vi "Main3.vi"() -> ()   [LabVIEW 2023]
uses:
  TEC LabVIEW Control Software v0.14/Source/LV Source/[meerstetter engineering TE Cooling]/TypeDefs/meTEC_ID 2000_Input Selection.ctl
  TEC LabVIEW Control Software v0.14/Source/LV Source/[meerstetter engineering TE Cooling]/TypeDefs/meTEC_ID 50011_Object Target Temperature Source Selection.ctl
  TEC LabVIEW Control Software v0.14/Source/LV Source/[meerstetter engineering TE Cooling]/TypeDefs/meTEC_ID 50000_Live Enable.ctl
  TEC LabVIEW Control Software v0.14/Source/LV Source/[meerstetter engineering TE Cooling]/TypeDefs/meTEC_ID 1200_Temperature is Stable.ctl
  TEC LabVIEW Control Software v0.14/Source/LV Source/[meerstetter engineering TE Cooling]/TypeDefs/meTEC_ID 104_Device Status.ctl
  Application_class/Instruments.ctl
  AD2_MSO_SDK_class/MSOConfig.ctl
  AD2_MSO_SDK_class/AD2TriggerSources.ctl
  AD2_MSO_SDK_class/MSORangeCh.ctl
  Application_class/Control 1.ctl
  Hamamatsu_class/SubRegion.ctl
  Application_class/Application.lvclass
  MTEC_Async_class/MTEC_Async.lvclass
  AD2andExtAWG_class/AD2andExtAWG.lvclass
  C:/GIT/PowerScan/InstrumentBase_class/AD2_SDK_class/InstrumentBase.lvclass
  <vilib>/Utility/error.llb/Error Cluster From Error Code.vi
  <vilib>/measure/matone.llb/Extract Single Tone Information 1 Chan.vi
  <vilib>/ErrorRing/Error Ring.xnode
  Hamamatsu_class/Hamamatsu.lvclass
  MTec_class/MTec.lvclass
  InstrumentBase_class/AD2_SDK_class/InstrumentBase.lvclass
  Experiment_class/Experiment.lvclass
  TDMSLogger_PowerScan_class/TDMSLogger_PowerScan.lvclass
  CetoniPump_class/CetoniPump.lvclass
  <vilib>/measure/NI_MAPro.lvlib
  AD2_MSO_SDK_class/AD2_MSO_SDK.lvclass
panel:
  in  "mem size":i32=100
  out "XY Graph":cluster{timestamp[], dbl[]}[](graph)=[{[timestamp(3810714974.4625654 s since 1904-01-01), timestamp(3810714974.6875706 s since 1904-01-01), timestamp(3810714974.9102407 s since 1904-01-01), timestamp(3810714975.132108 s since 1904-01-01), timestamp(3810714975.357173 s since 1904-01-01), timestamp(3810714975.581321 s since 1904-01-01), timestamp(3810714975.80342 s since 1904-01-01), timestamp(3810714976.0264726 s since 1904-01-01), timestamp(3810714976.250123 s since 1904-01-01), timestamp(3810714976.475124 s since 1904-01-01), timestamp(3810714976.6991234 s since 1904-01-01), timestamp(3810714976.9211745 s since 1904-01-01), timestamp(3810714977.1451674 s since 1904-01-01), timestamp(3810714977.368175 s since 1904-01-01), timestamp(3810714977.594176 s since 1904-01-01), timestamp(3810714977.816176 s since 1904-01-01), timestamp(3810714978.0411744 s since 1904-01-01), timestamp(3810714978.263168 s since 1904-01-01), timestamp(3810714978.488388 s since 1904-01-01), timestamp(3810714978.7113824 s since 1904-01-01), timestamp(3810714978.9333825 s since 1904-01-01), timestamp(3810714979.156552 s since 1904-01-01), timestamp(3810714979.380552 s since 1904-01-01), timestamp(3810714979.6040554 s since 1904-01-01), timestamp(3810714979.828112 s since 1904-01-01), timestamp(3810714980.051219 s since 1904-01-01), timestamp(3810714980.275273 s since 1904-01-01), timestamp(3810714980.499636 s since 1904-01-01), timestamp(3810714980.7226286 s since 1904-01-01), timestamp(3810714980.945965 s since 1904-01-01), timestamp(3810714981.170967 s since 1904-01-01), timestamp(3810714981.3933506 s since 1904-01-01), timestamp(3810714981.617357 s since 1904-01-01), timestamp(3810714981.840452 s since 1904-01-01), timestamp(3810714982.0654736 s since 1904-01-01), timestamp(3810714982.2894735 s since 1904-01-01), timestamp(3810714982.510492 s since 1904-01-01), timestamp(3810714982.734492 s since 1904-01-01), timestamp(3810714982.9584928 s since 1904-01-01), timestamp(3810714983.182848 s since 1904-01-01), timestamp(3810714983.4048495 s since 1904-01-01), timestamp(3810714983.6292033 s since 1904-01-01), timestamp(3810714983.8542337 s since 1904-01-01), timestamp(3810714984.077241 s since 1904-01-01), timestamp(3810714984.29924 s since 1904-01-01), timestamp(3810714984.52324 s since 1904-01-01), timestamp(3810714984.7462335 s since 1904-01-01), timestamp(3810714984.9702344 s since 1904-01-01), timestamp(3810714985.195372 s since 1904-01-01), timestamp(3810714985.417372 s since 1904-01-01), timestamp(3810714985.6413646 s since 1904-01-01), timestamp(3810714985.86677 s since 1904-01-01), timestamp(3810714986.0896926 s since 1904-01-01), timestamp(3810714986.311692 s since 1904-01-01), timestamp(3810714986.5356846 s since 1904-01-01), timestamp(3810714986.7598567 s since 1904-01-01), timestamp(3810714986.9828496 s since 1904-01-01), timestamp(3810714987.2071743 s since 1904-01-01), timestamp(3810714987.4291744 s since 1904-01-01), timestamp(3810714987.653329 s since 1904-01-01), timestamp(3810714987.8773217 s since 1904-01-01), timestamp(3810714988.1004457 s since 1904-01-01), timestamp(3810714988.325448 s since 1904-01-01), timestamp(3810714988.547662 s since 1904-01-01), timestamp(3810714988.7716546 s since 1904-01-01), timestamp(3810714988.994662 s since 1904-01-01), timestamp(3810714989.217661 s since 1904-01-01), timestamp(3810714989.443828 s since 1904-01-01), timestamp(3810714989.666828 s since 1904-01-01), timestamp(3810714989.890928 s since 1904-01-01), timestamp(3810714990.11292 s since 1904-01-01), timestamp(3810714990.335927 s since 1904-01-01), timestamp(3810714990.55996 s since 1904-01-01), timestamp(3810714990.7829666 s since 1904-01-01), timestamp(3810714991.006976 s since 1904-01-01), timestamp(3810714991.2310686 s since 1904-01-01), timestamp(3810714991.454176 s since 1904-01-01), timestamp(3810714991.679184 s since 1904-01-01), timestamp(3810714991.903184 s since 1904-01-01), timestamp(3810714992.125177 s since 1904-01-01), timestamp(3810714992.348177 s since 1904-01-01), timestamp(3810714992.572276 s since 1904-01-01), timestamp(3810714992.7962766 s since 1904-01-01), timestamp(3810714993.0195527 s since 1904-01-01), timestamp(3810714993.242547 s since 1904-01-01), timestamp(3810714993.4665465 s since 1904-01-01), timestamp(3810714993.6905394 s since 1904-01-01), timestamp(3810714993.913547 s since 1904-01-01), timestamp(3810714994.1385465 s since 1904-01-01), timestamp(3810714994.3625464 s since 1904-01-01), timestamp(3810714994.585547 s since 1904-01-01), timestamp(3810714994.80954 s since 1904-01-01), timestamp(3810714995.0335464 s since 1904-01-01), timestamp(3810714995.257552 s since 1904-01-01), timestamp(3810714995.4805474 s since 1904-01-01), timestamp(3810714995.7045465 s since 1904-01-01), timestamp(3810714995.925547 s since 1904-01-01), timestamp(3810714996.150547 s since 1904-01-01), timestamp(3810714996.374549 s since 1904-01-01), timestamp(3810714996.596541 s since 1904-01-01)], [22.902175903320312, 22.901992797851562, 22.903213500976562, 22.902908325195312, 22.903305053710938, 22.905197143554688, 22.906875610351562, 22.906539916992188, 22.906539916992188, 22.909378051757812, 22.910781860351562, 22.912826538085938, 22.915451049804688, 22.914047241210938, 22.917343139648438, 22.918472290039062, 22.918655395507812, 22.921981811523438, 22.920059204101562, 22.919723510742188, 22.918167114257812, 22.916549682617188, 22.915725708007812, 22.916458129882812, 22.916946411132812, 22.919662475585938, 22.916976928710938, 22.919906616210938, 22.921005249023438, 22.921249389648438, 22.922714233398438, 22.920883178710938, 22.924118041992188, 22.925735473632812, 22.928085327148438, 22.926986694335938, 22.929306030273438, 22.931716918945312, 22.930801391601562, 22.935470581054688, 22.936508178710938, 22.937179565429688, 22.939346313476562, 22.941116333007812, 22.940444946289062, 22.944534301757812, 22.943649291992188, 22.945999145507812, 22.944869995117188, 22.945846557617188, 22.945571899414062, 22.947494506835938, 22.948379516601562, 22.951004028320312, 22.948989868164062, 22.950271606445312, 22.950210571289062, 22.952072143554688, 22.951004028320312, 22.953475952148438, 22.954299926757812, 22.954116821289062, 22.953506469726562, 22.953598022460938, 22.954208374023438, 22.951828002929688, 22.953872680664062, 22.953018188476562, 22.953842163085938, 22.952865600585938, 22.955795288085938, 22.954513549804688, 22.955978393554688, 22.957351684570312, 22.954727172851562, 22.955886840820312, 22.955001831054688, 22.955825805664062, 22.954360961914062, 22.955032348632812, 22.957229614257812, 22.955490112304688, 22.958755493164062, 22.959518432617188, 22.959548950195312, 22.956710815429688, 22.959915161132812, 22.959487915039062, 22.959426879882812, 22.960617065429688, 22.960525512695312, 22.959243774414062, 22.960983276367188, 22.960647583007812, 22.962112426757812, 22.964004516601562, 22.964279174804688, 22.965377807617188, 22.964614868164062, 22.965621948242188]}, {[timestamp(3810714974.4625654 s since 1904-01-01), timestamp(3810714974.6875706 s since 1904-01-01), timestamp(3810714974.9102407 s since 1904-01-01), timestamp(3810714975.132108 s since 1904-01-01), timestamp(3810714975.357173 s since 1904-01-01), timestamp(3810714975.581321 s since 1904-01-01), timestamp(3810714975.80342 s since 1904-01-01), timestamp(3810714976.0264726 s since 1904-01-01), timestamp(3810714976.250123 s since 1904-01-01), timestamp(3810714976.475124 s since 1904-01-01), timestamp(3810714976.6991234 s since 1904-01-01), timestamp(3810714976.9211745 s since 1904-01-01), timestamp(3810714977.1451674 s since 1904-01-01), timestamp(3810714977.368175 s since 1904-01-01), timestamp(3810714977.594176 s since 1904-01-01), timestamp(3810714977.816176 s since 1904-01-01), timestamp(3810714978.0411744 s since 1904-01-01), timestamp(3810714978.263168 s since 1904-01-01), timestamp(3810714978.488388 s since 1904-01-01), timestamp(3810714978.7113824 s since 1904-01-01), timestamp(3810714978.9333825 s since 1904-01-01), timestamp(3810714979.156552 s since 1904-01-01), timestamp(3810714979.380552 s since 1904-01-01), timestamp(3810714979.6040554 s since 1904-01-01), timestamp(3810714979.828112 s since 1904-01-01), timestamp(3810714980.051219 s since 1904-01-01), timestamp(3810714980.275273 s since 1904-01-01), timestamp(3810714980.499636 s since 1904-01-01), timestamp(3810714980.7226286 s since 1904-01-01), timestamp(3810714980.945965 s since 1904-01-01), timestamp(3810714981.170967 s since 1904-01-01), timestamp(3810714981.3933506 s since 1904-01-01), timestamp(3810714981.617357 s since 1904-01-01), timestamp(3810714981.840452 s since 1904-01-01), timestamp(3810714982.0654736 s since 1904-01-01), timestamp(3810714982.2894735 s since 1904-01-01), timestamp(3810714982.510492 s since 1904-01-01), timestamp(3810714982.734492 s since 1904-01-01), timestamp(3810714982.9584928 s since 1904-01-01), timestamp(3810714983.182848 s since 1904-01-01), timestamp(3810714983.4048495 s since 1904-01-01), timestamp(3810714983.6292033 s since 1904-01-01), timestamp(3810714983.8542337 s since 1904-01-01), timestamp(3810714984.077241 s since 1904-01-01), timestamp(3810714984.29924 s since 1904-01-01), timestamp(3810714984.52324 s since 1904-01-01), timestamp(3810714984.7462335 s since 1904-01-01), timestamp(3810714984.9702344 s since 1904-01-01), timestamp(3810714985.195372 s since 1904-01-01), timestamp(3810714985.417372 s since 1904-01-01), timestamp(3810714985.6413646 s since 1904-01-01), timestamp(3810714985.86677 s since 1904-01-01), timestamp(3810714986.0896926 s since 1904-01-01), timestamp(3810714986.311692 s since 1904-01-01), timestamp(3810714986.5356846 s since 1904-01-01), timestamp(3810714986.7598567 s since 1904-01-01), timestamp(3810714986.9828496 s since 1904-01-01), timestamp(3810714987.2071743 s since 1904-01-01), timestamp(3810714987.4291744 s since 1904-01-01), timestamp(3810714987.653329 s since 1904-01-01), timestamp(3810714987.8773217 s since 1904-01-01), timestamp(3810714988.1004457 s since 1904-01-01), timestamp(3810714988.325448 s since 1904-01-01), timestamp(3810714988.547662 s since 1904-01-01), timestamp(3810714988.7716546 s since 1904-01-01), timestamp(3810714988.994662 s since 1904-01-01), timestamp(3810714989.217661 s since 1904-01-01), timestamp(3810714989.443828 s since 1904-01-01), timestamp(3810714989.666828 s since 1904-01-01), timestamp(3810714989.890928 s since 1904-01-01), timestamp(3810714990.11292 s since 1904-01-01), timestamp(3810714990.335927 s since 1904-01-01), timestamp(3810714990.55996 s since 1904-01-01), timestamp(3810714990.7829666 s since 1904-01-01), timestamp(3810714991.006976 s since 1904-01-01), timestamp(3810714991.2310686 s since 1904-01-01), timestamp(3810714991.454176 s since 1904-01-01), timestamp(3810714991.679184 s since 1904-01-01), timestamp(3810714991.903184 s since 1904-01-01), timestamp(3810714992.125177 s since 1904-01-01), timestamp(3810714992.348177 s since 1904-01-01), timestamp(3810714992.572276 s since 1904-01-01), timestamp(3810714992.7962766 s since 1904-01-01), timestamp(3810714993.0195527 s since 1904-01-01), timestamp(3810714993.242547 s since 1904-01-01), timestamp(3810714993.4665465 s since 1904-01-01), timestamp(3810714993.6905394 s since 1904-01-01), timestamp(3810714993.913547 s since 1904-01-01), timestamp(3810714994.1385465 s since 1904-01-01), timestamp(3810714994.3625464 s since 1904-01-01), timestamp(3810714994.585547 s since 1904-01-01), timestamp(3810714994.80954 s since 1904-01-01), timestamp(3810714995.0335464 s since 1904-01-01), timestamp(3810714995.257552 s since 1904-01-01), timestamp(3810714995.4805474 s since 1904-01-01), timestamp(3810714995.7045465 s since 1904-01-01), timestamp(3810714995.925547 s since 1904-01-01), timestamp(3810714996.150547 s since 1904-01-01), timestamp(3810714996.374549 s since 1904-01-01), timestamp(3810714996.596541 s since 1904-01-01)], [23.093063354492188, 23.094924926757812, 23.094497680664062, 23.097518920898438, 23.095504760742188, 23.094528198242188, 23.098098754882812, 23.099533081054688, 23.102035522460938, 23.100082397460938, 23.105026245117188, 23.107894897460938, 23.107254028320312, 23.108169555664062, 23.112472534179688, 23.110580444335938, 23.116165161132812, 23.113418579101562, 23.113418579101562, 23.112075805664062, 23.110916137695312, 23.108871459960938, 23.107559204101562, 23.110641479492188, 23.111648559570312, 23.111618041992188, 23.113174438476562, 23.115737915039062, 23.115188598632812, 23.116897583007812, 23.113906860351562, 23.116683959960938, 23.119857788085938, 23.119705200195312, 23.120559692382812, 23.123886108398438, 23.123031616210938, 23.122512817382812, 23.124221801757812, 23.128158569335938, 23.127243041992188, 23.129959106445312, 23.131637573242188, 23.131820678710938, 23.133285522460938, 23.136337280273438, 23.136276245117188, 23.136917114257812, 23.138320922851562, 23.137313842773438, 23.141921997070312, 23.142196655273438, 23.142440795898438, 23.143112182617188, 23.145858764648438, 23.144485473632812, 23.147598266601562, 23.147171020507812, 23.149276733398438, 23.149337768554688, 23.149276733398438, 23.152023315429688, 23.155258178710938, 23.155410766601562, 23.153366088867188, 23.155471801757812, 23.154800415039062, 23.155899047851562, 23.157669067382812, 23.159255981445312, 23.157211303710938, 23.157821655273438, 23.160781860351562, 23.162673950195312, 23.161300659179688, 23.164657592773438, 23.164108276367188, 23.163711547851562, 23.162490844726562, 23.165390014648438, 23.165481567382812, 23.165939331054688, 23.165573120117188, 23.169692993164062, 23.168869018554688, 23.167984008789062, 23.168258666992188, 23.168411254882812, 23.168258666992188, 23.168899536132812, 23.170425415039062, 23.170089721679688, 23.171829223632812, 23.173904418945312, 23.172744750976562, 23.175460815429688, 23.173141479492188, 23.174606323242188, 23.174728393554688, 23.175674438476562]}, {[timestamp(3810714974.4625654 s since 1904-01-01), timestamp(3810714974.6875706 s since 1904-01-01), timestamp(3810714974.9102407 s since 1904-01-01), timestamp(3810714975.132108 s since 1904-01-01), timestamp(3810714975.357173 s since 1904-01-01), timestamp(3810714975.581321 s since 1904-01-01), timestamp(3810714975.80342 s since 1904-01-01), timestamp(3810714976.0264726 s since 1904-01-01), timestamp(3810714976.250123 s since 1904-01-01), timestamp(3810714976.475124 s since 1904-01-01), timestamp(3810714976.6991234 s since 1904-01-01), timestamp(3810714976.9211745 s since 1904-01-01), timestamp(3810714977.1451674 s since 1904-01-01), timestamp(3810714977.368175 s since 1904-01-01), timestamp(3810714977.594176 s since 1904-01-01), timestamp(3810714977.816176 s since 1904-01-01), timestamp(3810714978.0411744 s since 1904-01-01), timestamp(3810714978.263168 s since 1904-01-01), timestamp(3810714978.488388 s since 1904-01-01), timestamp(3810714978.7113824 s since 1904-01-01), timestamp(3810714978.9333825 s since 1904-01-01), timestamp(3810714979.156552 s since 1904-01-01), timestamp(3810714979.380552 s since 1904-01-01), timestamp(3810714979.6040554 s since 1904-01-01), timestamp(3810714979.828112 s since 1904-01-01), timestamp(3810714980.051219 s since 1904-01-01), timestamp(3810714980.275273 s since 1904-01-01), timestamp(3810714980.499636 s since 1904-01-01), timestamp(3810714980.7226286 s since 1904-01-01), timestamp(3810714980.945965 s since 1904-01-01), timestamp(3810714981.170967 s since 1904-01-01), timestamp(3810714981.3933506 s since 1904-01-01), timestamp(3810714981.617357 s since 1904-01-01), timestamp(3810714981.840452 s since 1904-01-01), timestamp(3810714982.0654736 s since 1904-01-01), timestamp(3810714982.2894735 s since 1904-01-01), timestamp(3810714982.510492 s since 1904-01-01), timestamp(3810714982.734492 s since 1904-01-01), timestamp(3810714982.9584928 s since 1904-01-01), timestamp(3810714983.182848 s since 1904-01-01), timestamp(3810714983.4048495 s since 1904-01-01), timestamp(3810714983.6292033 s since 1904-01-01), timestamp(3810714983.8542337 s since 1904-01-01), timestamp(3810714984.077241 s since 1904-01-01), timestamp(3810714984.29924 s since 1904-01-01), timestamp(3810714984.52324 s since 1904-01-01), timestamp(3810714984.7462335 s since 1904-01-01), timestamp(3810714984.9702344 s since 1904-01-01), timestamp(3810714985.195372 s since 1904-01-01), timestamp(3810714985.417372 s since 1904-01-01), timestamp(3810714985.6413646 s since 1904-01-01), timestamp(3810714985.86677 s since 1904-01-01), timestamp(3810714986.0896926 s since 1904-01-01), timestamp(3810714986.311692 s since 1904-01-01), timestamp(3810714986.5356846 s since 1904-01-01), timestamp(3810714986.7598567 s since 1904-01-01), timestamp(3810714986.9828496 s since 1904-01-01), timestamp(3810714987.2071743 s since 1904-01-01), timestamp(3810714987.4291744 s since 1904-01-01), timestamp(3810714987.653329 s since 1904-01-01), timestamp(3810714987.8773217 s since 1904-01-01), timestamp(3810714988.1004457 s since 1904-01-01), timestamp(3810714988.325448 s since 1904-01-01), timestamp(3810714988.547662 s since 1904-01-01), timestamp(3810714988.7716546 s since 1904-01-01), timestamp(3810714988.994662 s since 1904-01-01), timestamp(3810714989.217661 s since 1904-01-01), timestamp(3810714989.443828 s since 1904-01-01), timestamp(3810714989.666828 s since 1904-01-01), timestamp(3810714989.890928 s since 1904-01-01), timestamp(3810714990.11292 s since 1904-01-01), timestamp(3810714990.335927 s since 1904-01-01), timestamp(3810714990.55996 s since 1904-01-01), timestamp(3810714990.7829666 s since 1904-01-01), timestamp(3810714991.006976 s since 1904-01-01), timestamp(3810714991.2310686 s since 1904-01-01), timestamp(3810714991.454176 s since 1904-01-01), timestamp(3810714991.679184 s since 1904-01-01), timestamp(3810714991.903184 s since 1904-01-01), timestamp(3810714992.125177 s since 1904-01-01), timestamp(3810714992.348177 s since 1904-01-01), timestamp(3810714992.572276 s since 1904-01-01), timestamp(3810714992.7962766 s since 1904-01-01), timestamp(3810714993.0195527 s since 1904-01-01), timestamp(3810714993.242547 s since 1904-01-01), timestamp(3810714993.4665465 s since 1904-01-01), timestamp(3810714993.6905394 s since 1904-01-01), timestamp(3810714993.913547 s since 1904-01-01), timestamp(3810714994.1385465 s since 1904-01-01), timestamp(3810714994.3625464 s since 1904-01-01), timestamp(3810714994.585547 s since 1904-01-01), timestamp(3810714994.80954 s since 1904-01-01), timestamp(3810714995.0335464 s since 1904-01-01), timestamp(3810714995.257552 s since 1904-01-01), timestamp(3810714995.4805474 s since 1904-01-01), timestamp(3810714995.7045465 s since 1904-01-01), timestamp(3810714995.925547 s since 1904-01-01), timestamp(3810714996.150547 s since 1904-01-01), timestamp(3810714996.374549 s since 1904-01-01), timestamp(3810714996.596541 s since 1904-01-01)], [0.0, 0.0, 0.0, 0.0, 0.0, 0.0, 0.0, 0.0, 0.0, 0.0, 0.0, 0.0, 0.0, 0.0, 0.0, 0.0, 0.0, 0.0, 0.0, 0.0, 0.0, 0.0, 0.0, 0.0, 0.0, 0.0, 0.0, 0.0, 0.0, 0.0, 0.0, 0.0, 0.0, 0.0, 0.0, 0.0, 0.0, 0.0, 0.0, 0.0, 0.0, 0.0, 0.0, 0.0, 0.0, 0.0, 0.0, 0.0, 0.0, 0.0, 0.0, 0.0, 0.0, 0.0, 0.0, 0.0, 0.0, 0.0, 0.0, 0.0, 0.0, 0.0, 0.0, 0.0, 0.0, 0.0, 0.0, 0.0, 0.0, 0.0, 0.0, 0.0, 0.0, 0.0, 0.0, 0.0, 0.0, 0.0, 0.0, 0.0, 0.0, 0.0, 0.0, 0.0, 0.0, 0.0, 0.0, 0.0, 0.0, 0.0, 0.0, 0.0, 0.0, 0.0, 0.0, 0.0, 0.0, 0.0, 0.0, 0.0]}]
  in  "Chart Length":enum16{"60 s", "10 minutes", "1 h"}(ring)=enum."10 minutes"
  out "Waveform Chart":waveform(dbl)[](graph)=[{"t0"=timestamp(3810714996.596541 s since 1904-01-01), "dt"=1.0, "Y"=[22.965621948242188]}, {"t0"=timestamp(3810714996.596541 s since 1904-01-01), "dt"=1.0, "Y"=[23.175674438476562]}]
  in  "Read MSO":bool
  out "error out":errorcluster
  out "Status":string="Exiting.."
  in  "AutoScaleCh1":bool=TRUE caption="AutoScale timebase to ChA"
  out "V/Hz/Deg":dbl[](array[numeric])=[256495.2123849432, 0.012104949851784449, 127.31074154871095, 4268838.632377055, 0.0003381910830981614, 134.9693104826537]
  out "Data":string[](array[string])=["Ch1Freq", "Ch1Amp", "Ch1Phase", "Ch2Freq", "Ch2Amp", "Ch2Phase"]
  out "MSO Data WaveForms 2":waveform(dbl)[](graph)=[{"t0"=timestamp(0 s since 1904-01-01), "dt"=1e-08, "Y"=array[8192 elements]}, {"t0"=timestamp(0 s since 1904-01-01), "dt"=1e-08, "Y"=array[8192 elements]}]
  in  "ABORT":bool
  in  "Tab Control":T1(tab)=enum."Cetoni"
  in  "Use Cetoni?":bool=TRUE
  in  "Use Hamamatsu":bool=TRUE
  in  "Use MeTEC?":bool=TRUE
  in  "AWG VISA resource name":refnum<visa-resource-name>="USB0::0x0699::0x0347::C037907::INSTR"
  in  "System Configuration":T2
  in  "Initialize System":bool
  in  "Use Instruments?":bool=TRUE
  in  "Device Configuration Path":string="C:\\Users\\Public\\Documents\\QmixElements\\Projects\\default_project\\Configurations\\double"
  in  "Turn Off WFG During Refill":bool
  in  "index":i32
  in  "refill below level(uL)":dbl=1000.0
  in  "Refill":bool
  in  "Conditional Refill":bool
  in  "Empty":bool
  in  "Stop pumps":bool
  in  "SyringeSettings":T3={"Maximum Piston Stroke (mm)"=66.0, "Inner Diameter (mm)"=14.5}
  in  "Configure Syringe":bool
  in  "ValveControl":cluster{"index":i32, "Valve Position":bool}
  in  "Go to Level":bool
  in  "GoToLevelSettings":T4={"index"=0, "Level(uL)"=0.0, "Flow"=250.0}
  in  "Monitor Pump":bool
  out "Array":T5(array[cluster])=[{"Pump Name"="neMESYS_Low_Pressure_1_Pump", "Actual Flow Rate"=249.9994261659258, "Fill Level"=9609.141943854513, "Is pumping"=TRUE}, {"Pump Name"="neMESYS_Low_Pressure_2_Pump", "Actual Flow Rate"=0.0, "Fill Level"=0.0, "Is pumping"=FALSE}]
  in  "ReferenceMove":bool
  in  "refill and \nempty rate(uL/min)":dbl=12000.0
  out "Cluster":T8={"meTEC_CH2_Temperature Stability"=0, "meTEC_CH2_Act. Output Current [A]"=0.009997940622270107, "meTEC_CH2_Act. Output Voltage [V]"=0.004072710871696472, "meTEC_CH2_Object Temperature [°C]"=23.175674438476562, "meTEC_CH2_Sink Temperature [°C]"=25.0, "meTEC_CH1_Error Parameter"=0, "meTEC_CH1_Error Instance"=0, "meTEC_CH1_Error No."=0, "meTEC_CH1_Device Status"=1, "meTEC_CH1_Temperature Stability"=0, "meTEC_CH1_Act. Output Current [A]"=0.010120010934770107, "meTEC_CH1_Act. Output Voltage [V]"=0.009891997091472149, "meTEC_CH1_Object Temperature [°C]"=22.965621948242188, "meTEC_CH1_Sink Temperature [°C]"=25.0} {"meTEC_CH1_Sink Temperature [°C]" format="%.3f"; "meTEC_CH1_Object Temperature [°C]" format="%.3f"; "meTEC_CH1_Act. Output Voltage [V]" format="%.3f"; "meTEC_CH1_Act. Output Current [A]" format="%.3f"; "meTEC_CH1_Temperature Stability" items=["Temperature regulation is not active", "Is not stable", "Is stable"]; "meTEC_CH1_Device Status" items=["Initializing", "Ready", "Run", "Error", "Bootloader", "Reset in Progress"]; "meTEC_CH2_Sink Temperature [°C]" format="%.3f"; "meTEC_CH2_Object Temperature [°C]" format="%.3f"; "meTEC_CH2_Act. Output Voltage [V]" format="%.3f"; "meTEC_CH2_Act. Output Current [A]" format="%.3f"; "meTEC_CH2_Temperature Stability" items=["Temperature regulation is not active", "Is not stable", "Is stable"]}
  in  "Config Data":T12={"meTEC_CH1_Input Selection (ID 2000)"=2, "meTEC_CH2_Input Selection (ID 2000)"=2, "meTEC_CH1_Object Target Temp. Source Selection (ID 50011)"=0, "meTEC_CH2_Object Target Temp. Source Selection (ID 50011)"=0, "meTEC_CH1_Live Enable (ID 50000)"=0, "meTEC_CH2_Live Enable (ID 50000)"=0, "meTEC_CH1_Object Target Temperature (ID 3000 / 50012) [°C]"=23.0, "meTEC_CH2_Object Target Temperature (ID 3000 / 50012) [°C]"=23.0, "meTEC_CH1_Live Set Current (ID 50001) [A]"=0.0, "meTEC_CH2_Live Set Current (ID 50001) [A]"=0.0, "meTEC_CH1_Live Set Voltage (ID 50002) [V]"=0.0, "meTEC_CH2_Live Set Voltage (ID 50002) [V]"=0.0} {"meTEC_CH2_Live Set Voltage (ID 50002) [V]" format="%#.3f"; "meTEC_CH1_Live Set Voltage (ID 50002) [V]" format="%#.3f"; "meTEC_CH2_Live Set Current (ID 50001) [A]" format="%#.3f"; "meTEC_CH1_Live Set Current (ID 50001) [A]" format="%#.3f"; "meTEC_CH2_Object Target Temperature (ID 3000 / 50012) [°C]" format="%#.3f"; "meTEC_CH1_Object Target Temperature (ID 3000 / 50012) [°C]" format="%#.3f"; "meTEC_CH2_Live Enable (ID 50000)" items=["Disabled (Reset State)", "Enabled"]; "meTEC_CH1_Live Enable (ID 50000)" items=["Disabled (Reset State)", "Enabled"]; "meTEC_CH2_Object Target Temp. Source Selection (ID 50011)" items=["Parameter ID 3000 (Reset State)", "Parameter ID 50012"]; "meTEC_CH1_Object Target Temp. Source Selection (ID 50011)" items=["Parameter ID 3000 (Reset State)", "Parameter ID 50012"]; "meTEC_CH2_Input Selection (ID 2000)" items=["Static Current / Voltage", "Live Current / Voltage", "Temperature Controller"]; "meTEC_CH1_Input Selection (ID 2000)" items=["Static Current / Voltage", "Live Current / Voltage", "Temperature Controller"]}
  in  "Configure TEC":bool
  in  "Monitor":bool=TRUE
  in  "ResetMtec":bool
  in  "Metec Flush Memory":bool
  in  "OutputEnable":T13
  in  "Config WFG":bool
  in  "Freq Ch1&2":T14
  in  "Configdatastd":T15={"ConfigDataCh1"={"Frequency Hz (1000 Hz)"=1000.0, "Waveform Function (0: Sine)"=0, "Amplitude (1 Vpp)"=1.0, "DC Offset (0.00 V)"=0.0, "Phase Level (-1)"=0.0, "Phase Unit (0: Radian)"=0}, "ConfigDataCh2"={"Frequency Hz (1000 Hz)"=1000.0, "Waveform Function (0: Sine)"=0, "Amplitude (1 Vpp)"=1.0, "DC Offset (0.00 V)"=0.0, "Phase Level (-1)"=0.0, "Phase Unit (0: Radian)"=0}} {"ConfigDataCh1"."Frequency Hz (1000 Hz)" min=0.0 max=100000000.0}
  in  "CurrentProbeScaling(V/A)":dbl=5.0
  in  "PwrScanSettings":T16={"FreqStart(Hz)"=1800000.0, "Increment(Hz)"=1000.0, "Steps"=100}
  out "Power Graph":T17=[{"PwrFreq"=[1800000.0, 1801000.0, 1802000.0, 1803000.0, 1804000.0, 1805000.0, 1806000.0, 1807000.0, 1808000.0, 1809000.0, 1810000.0, 1811000.0, 1812000.0, 1813000.0, 1814000.0, 1815000.0, 1816000.0, 1817000.0, 1818000.0, 1819000.0, 1820000.0, 1821000.0, 1822000.0, 1823000.0, 1824000.0, 1825000.0, 1826000.0, 1827000.0, 1828000.0, 1829000.0, 1830000.0, 1831000.0, 1832000.0, 1833000.0, 1834000.0, 1835000.0, 1836000.0, 1837000.0, 1838000.0, 1839000.0, 1840000.0, 1841000.0, 1842000.0, 1843000.0, 1844000.0, 1845000.0, 1846000.0, 1847000.0, 1848000.0, 1849000.0, 1850000.0, 1851000.0, 1852000.0, 1853000.0, 1854000.0, 1855000.0, 1856000.0, 1857000.0, 1858000.0, 1859000.0, 1860000.0, 1861000.0, 1862000.0, 1863000.0, 1864000.0, 1865000.0, 1866000.0, 1867000.0, 1868000.0, 1869000.0, 1870000.0, 1871000.0, 1872000.0, 1873000.0, 1874000.0, 1875000.0, 1876000.0, 1877000.0, 1878000.0, 1879000.0, 1880000.0, 1881000.0, 1882000.0, 1883000.0, 1884000.0, 1885000.0, 1886000.0, 1887000.0, 1888000.0, 1889000.0, 1890000.0, 1891000.0, 1892000.0, 1893000.0, 1894000.0, 1895000.0, 1896000.0, 1897000.0, 1898000.0, 1899000.0], "PwrMeasured"=[0.03743018699905172, 0.03868842711054406, 0.039939450983681936, 0.041186940846945984, 0.042492363236693975, 0.04404846555067622, 0.04602835102242353, 0.04843888820937301, 0.05119026075250401, 0.054137745072059686, 0.05681989848669318, 0.05866977349663312, 0.05974650294953525, 0.06005376515825572, 0.05994285605916934, 0.05965859181003201, 0.05940789816848652, 0.05911436810870655, 0.05887115083576992, 0.058285278937152116, 0.05733209401753114, 0.05612065814579392, 0.05491201122450486, 0.054246204884069796, 0.05413387963390649, 0.0544784492868222, 0.055223443274043806, 0.05584761484864832, 0.05593777472478643, 0.055604310692913786, 0.05518644597062401, 0.054618464862787694, 0.054214223715299915, 0.05394256784700533, 0.0538322569007853, 0.05378224385812821, 0.053684397213232725, 0.053570515853526054, 0.05367988225271155, 0.05367731285637497, 0.05328103475935342, 0.05261733484260826, 0.05172095371283941, 0.050922021343682664, 0.05021598202266246, 0.049693559571941236, 0.04964157824916153, 0.049770317527984026, 0.04982229343352004, 0.0491940448801376, 0.048088239496034246, 0.0465169483544214, 0.0449815088404273, 0.04339710247015175, 0.04200318845517933, 0.04079371088999795, 0.03986802195324547, 0.038792483453571246, 0.03777766173772913, 0.03677527534117768, 0.0359760414327305, 0.03518671210489007, 0.03475002270949958, 0.03471532342952112, 0.03517735874853088, 0.03613562839997322, 0.0377065106935801, 0.0398207089338458, 0.04192610453201364, 0.04433368155489899, 0.04724045693183674, 0.05041187326865423, 0.05357414254285915, 0.056935687754456586, 0.06034831631771629, 0.06370638524387114, 0.06689701401467622, 0.06907501466358135, 0.07011171729016413, 0.06928919978057443, 0.06697831206028507, 0.06356111518422408, 0.059707919276213384, 0.055820271940164715, 0.05201579594450088, 0.048220123240964884, 0.044549547433591366, 0.04117661978432694, 0.038128405762736364, 0.03561051707739825, 0.03331342696116638, 0.03141526136270806, 0.029497507637866037, 0.02786984120696333, 0.0266553633197663, 0.025619681037449903, 0.024768741920820493, 0.024028995090048973, 0.023324807778494015, 0.022671870223729386]}, {"PwrFreq"=[], "PwrMeasured"=[]}, {"PwrFreq"=[], "PwrMeasured"=[]}]
  in  "AdjustPower":bool
  in  "DesiredPower(W)":dbl=0.001 min=0.001
  out "min Power":dbl=0.022671870223729386
  out "max Power":dbl=0.07011171729016413
  out "Measured Power":dbl=0.014358194668451557
  in  "MeasurePower":bool
  out "AmplitudeOk":bool=TRUE
  in  "Run Power Scan":bool
  out "phase (deg)":dbl=82.9743375382008
  out "impedance (ohm)":dbl=0.07240014859741192
  in  "Config":T18={"Timing"={"Enable"=TRUE, "Samples In"=8000.0, "Sample Rate"=100000000.0, "Mode"=enum."Single Sample"}, "Trigger"={"Hysteresis"=0.0, "Trigger Level"=0.0, "Trigger Condition"=0, "Trigger Type"=0, "Trigger Channel"=0, "secTimeout"=0.5, "TrigrSrc"=enum."trigsrcDetectorAnalogIn"}, "Range Ch1"={"idxChannel"=0, "voltOffset"=0.0, "VoltsRange"=50}, "Range Ch 2"={"idxChannel"=1, "voltOffset"=0.0, "VoltsRange"=5}} {"Range Ch 2"."VoltsRange" items=["High 50V"=50, "Low5V"=5]; "Range Ch1"."VoltsRange" items=["High 50V"=50, "Low5V"=5]; "Trigger"."Trigger Channel" items=["Channel 1"=0, "Channel 2"=1, "Both"=-1]; "Trigger"."Trigger Type" items=["Edge", "Pulse", "Transition"]; "Trigger"."Trigger Condition" items=["Rising", "Falling"]}
  in  "Configure MSO":bool
  in  "AutoRange MSO (Volt)":bool
  in  "Center ROI":bool=TRUE
  in  "Image":bool
  in  "Image Continous":bool
  in  "ExposureTime(ms)":dbl=5.0
  in  "ROI":T21={"Horizontal Offset"=0, "Vertical Offset"=652, "Horizontal Size"=2304, "Vertical Size"=1000} {"Vertical Size" min=4 max=1652 step=4; "Horizontal Size" min=4 max=2304 step=4; "Vertical Offset" min=0 max=1304 step=4; "Horizontal Offset" min=0 max=0 step=4}
  in  "Configure":bool
  in  "Fill List":bool
  in  "Number of Frequencies":dbl=101.0
  in  "Freq Increment":dbl=1000.0
  in  "Freq Start":dbl=1800000.0
  in  "Start Experiment":bool
  in  "Number of Images (#)":i32=10
  in  "wait time(s)":dbl
  in  "List of Powers to run(W)":dbl[](array[numeric])=[0.01, 0.02] min=0.001
  in  "List of Frequencies (Hz)":dbl[](array[numeric])=[1800000.0, 1801000.0, 1802000.0, 1803000.0, 1804000.0, 1805000.0, 1806000.0, 1807000.0, 1808000.0, 1809000.0, 1810000.0, 1811000.0, 1812000.0, 1813000.0, 1814000.0, 1815000.0, 1816000.0, 1817000.0, 1818000.0, 1819000.0, 1820000.0, 1821000.0, 1822000.0, 1823000.0, 1824000.0, 1825000.0, 1826000.0, 1827000.0, 1828000.0, 1829000.0, 1830000.0, 1831000.0, 1832000.0, 1833000.0, 1834000.0, 1835000.0, 1836000.0, 1837000.0, 1838000.0, 1839000.0, 1840000.0, 1841000.0, 1842000.0, 1843000.0, 1844000.0, 1845000.0, 1846000.0, 1847000.0, 1848000.0, 1849000.0, 1850000.0, 1851000.0, 1852000.0, 1853000.0, 1854000.0, 1855000.0, 1856000.0, 1857000.0, 1858000.0, 1859000.0, 1860000.0, 1861000.0, 1862000.0, 1863000.0, 1864000.0, 1865000.0, 1866000.0, 1867000.0, 1868000.0, 1869000.0, 1870000.0, 1871000.0, 1872000.0, 1873000.0, 1874000.0, 1875000.0, 1876000.0, 1877000.0, 1878000.0, 1879000.0, 1880000.0, 1881000.0, 1882000.0, 1883000.0, 1884000.0, 1885000.0, 1886000.0, 1887000.0, 1888000.0, 1889000.0, 1890000.0, 1891000.0, 1892000.0, 1893000.0, 1894000.0, 1895000.0, 1896000.0, 1897000.0, 1898000.0, 1899000.0, 1900000.0] min=0.001
  out "Progress (100%)":dbl=100.0
  in  "List of Flow Rates (ul/min)":dbl[](array[numeric])=[250.0]
  out "# elements in queue":i32=3256
  in  "Repeat Adjust Power and Wait N Times (#)":i32=1 min=1
  in  "wait after adjust power (s)":dbl
  in  "wait after changing flow rate(s)":dbl
  in  "AutoRange MSO":bool
  in  "Exit":bool
  # "All Power Levels"
  # "All Frequencies"
  # "All Flow Rates"
  # "Conditional Refill\nSet Flow\nChange Frequency\nEnable Function Generator\nAdjust Power\nWait (Adjust Power)\nWait\nSave Data (N times)\nDisable Function Generator\nWait\nSave Data"
  # "Measured Waveform"
  # "Index of the pump you are controlling"
  # "This one goes to 11!"
  # "Refills if syringe\nis below level"
  # "(sets it back to its previous state after)"
  # "Volt on ch1 and Current Probe ch2"
  # "(also measures impedance)"
  # "All Power Levels"
  # "All Frequencies"
  # "All Flow Rates"
  # "Conditional Refill\nSet Flow\nWait (flow)\nChange Frequency\nEnable Function Generator\nAdjust Power\nWait (Adjust Power)\nWait\nSave Data (N times)\nDisable Function Generator\nWait\nSave Data"
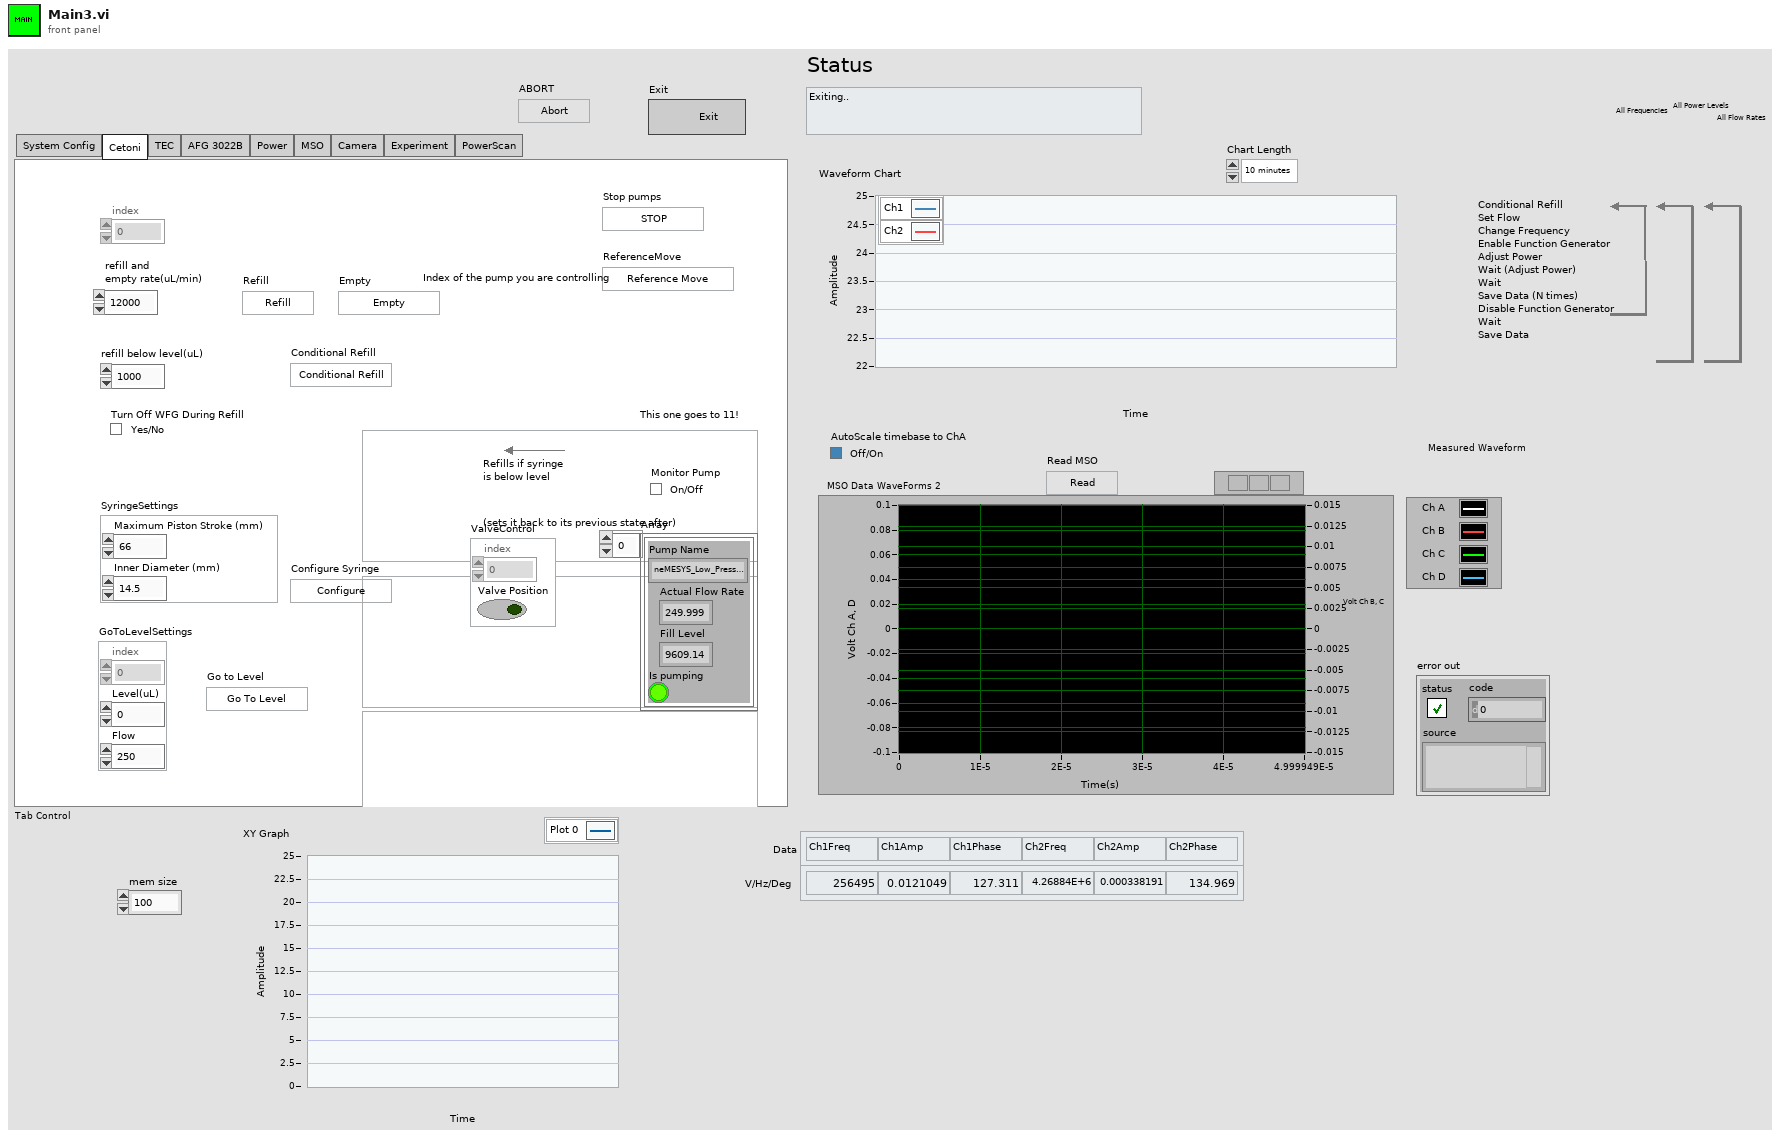
[diagram p1: front panel]
types:
  T1 = enum32{"System Config", "Cetoni", "TEC", "AFG 3022B", "Power", "MSO", "Camera", "Experiment", "PowerScan"}
  T2 = typedef "Application.lvclass/Instruments.ctl" = enum16{"AD2 and AFG3022"}
  T3 = cluster{"Maximum Piston Stroke (mm)":dbl, "Inner Diameter (mm)":dbl}
  T4 = cluster{"index":i32, "Level(uL)":dbl, "Flow":dbl}
  T5 = cluster{"Pump Name":string, "Actual Flow Rate":dbl, "Fill Level":dbl, "Is pumping":bool}[]
  T6 = typedef "meTEC_ID 1200_Temperature is Stable.ctl" = i32
  T7 = typedef "meTEC_ID 104_Device Status.ctl" = i32
  T8 = cluster{"meTEC_CH2_Temperature Stability":T6, "meTEC_CH2_Act. Output Current [A]":dbl, "meTEC_CH2_Act. Output Voltage [V]":dbl, "meTEC_CH2_Object Temperature [°C]":dbl, "meTEC_CH2_Sink Temperature [°C]":dbl, "meTEC_CH1_Error Parameter":i32, "meTEC_CH1_Error Instance":i32, "meTEC_CH1_Error No.":i32, "meTEC_CH1_Device Status":T7, "meTEC_CH1_Temperature Stability":T6, "meTEC_CH1_Act. Output Current [A]":dbl, "meTEC_CH1_Act. Output Voltage [V]":dbl, "meTEC_CH1_Object Temperature [°C]":dbl, "meTEC_CH1_Sink Temperature [°C]":dbl}
  T9 = typedef "meTEC_ID 2000_Input Selection.ctl" = i32
  T10 = typedef "meTEC_ID 50011_Object Target Temperature Source Selection.ctl" = i32
  T11 = typedef "meTEC_ID 50000_Live Enable.ctl" = i32
  T12 = cluster{"meTEC_CH1_Input Selection (ID 2000)":T9, "meTEC_CH2_Input Selection (ID 2000)":T9, "meTEC_CH1_Object Target Temp. Source Selection (ID 50011)":T10, "meTEC_CH2_Object Target Temp. Source Selection (ID 50011)":T10, "meTEC_CH1_Live Enable (ID 50000)":T11, "meTEC_CH2_Live Enable (ID 50000)":T11, "meTEC_CH1_Object Target Temperature (ID 3000 / 50012) [°C]":dbl, "meTEC_CH2_Object Target Temperature (ID 3000 / 50012) [°C]":dbl, "meTEC_CH1_Live Set Current (ID 50001) [A]":dbl, "meTEC_CH2_Live Set Current (ID 50001) [A]":dbl, "meTEC_CH1_Live Set Voltage (ID 50002) [V]":dbl, "meTEC_CH2_Live Set Voltage (ID 50002) [V]":dbl}
  T13 = cluster{"Enable Output WFG Ch1":bool, "Enable Output WFG Ch 2":bool}
  T14 = cluster{"Ch1.Carrier.Frequency (Hz)":dbl, "Ch2.Carrier.Frequency (Hz)":dbl}
  T15 = cluster{"ConfigDataCh1":cluster{"Frequency Hz (1000 Hz)":dbl, "Waveform Function (0: Sine)":u16, "Amplitude (1 Vpp)":dbl, "DC Offset (0.00 V)":dbl, "Phase Level (-1)":dbl, "Phase Unit (0: Radian)":u16}, "ConfigDataCh2":cluster{"Frequency Hz (1000 Hz)":dbl, "Waveform Function (0: Sine)":u16, "Amplitude (1 Vpp)":dbl, "DC Offset (0.00 V)":dbl, "Phase Level (-1)":dbl, "Phase Unit (0: Radian)":u16}}
  T16 = cluster{"FreqStart(Hz)":dbl, "Increment(Hz)":dbl, "Steps":i32}
  T17 = typedef "Control 1.ctl" = cluster{"PwrFreq":dbl[], "PwrMeasured":dbl[]}[]
  T18 = typedef "AD2_MSO_SDK.lvclass/MSOConfig.ctl" = cluster{"Timing":cluster{"Enable":bool, "Samples In":dbl, "Sample Rate":dbl, "Mode":enum16{"Single Sample", "Scanshift", "Multiple Samples", "Scan Screen"}}, "Trigger":cluster{"Hysteresis":dbl, "Trigger Level":dbl, "Trigger Condition":i32, "Trigger Type":i32, "Trigger Channel":i32, "secTimeout":dbl, "TrigrSrc":T19}, "Range Ch1":T20, "Range Ch 2":T20}
  T19 = typedef "AD2_MSO_SDK.lvclass/AD2TriggerSources.ctl" = enum8{"trigrsrcNone", "trigsrcPC", "trigsrcDetectorAnalogIn", "trigsrcDetectorDigitalIn", "trigsrcAnalogIn", "trigsrcDigitalIn", "trigsrcDigitalOut", "trigsrcAnalogOut1", "trigsrcAnalogOut2", "trigsrcAnalogOut3", "trigsrcAnalogOut4", "trigsrcExternal1", "trigsrcExternal2", "trigsrcExternal3", "trigsrcExternal4", ""}
  T20 = typedef "AD2_MSO_SDK.lvclass/MSORangeCh.ctl" = cluster{"idxChannel":i32, "voltOffset":dbl, "VoltsRange":u16}
  T21 = typedef "Hamamatsu.lvclass/SubRegion.ctl" = cluster{"Horizontal Offset":i32, "Vertical Offset":i32, "Horizontal Size":i32, "Vertical Size":i32}
  T22 = cluster{"index":i32, "Level(ml)":dbl, "Flow":dbl}
  T23 = typedef "LVMinMaxIncTypeDef.ctl" = cluster{"Minimum":dbl, "Maximum":dbl, "Increment":dbl}
  T24 = cluster{"H Offset":cluster{"Value":i32, "Limits":T23}, "V Offset":cluster{"Value":i32, "Limits":T23}, "H Size":cluster{"Value":i32, "Limits":T23}, "V Size":cluster{"Value":i32, "Limits":T23}}
  T25 = typedef "Hamamatsu.lvclass/SubRegionLimits.ctl" = cluster{"H Offset":cluster{"Value":i32, "Limits":T23}, "V Offset":cluster{"Value":i32, "Limits":T23}, "H Size":cluster{"Value":i32, "Limits":T23}, "V Size":cluster{"Value":i32, "Limits":T23}}
  T26 = typedef "IMAQ Image.ctl" = refnum<image>
  T27 = cluster{"current time":timestamp, "DataOut":cluster{"meTEC_CH2_Temperature Stability":T6, "meTEC_CH2_Act. Output Current [A]":dbl, "meTEC_CH2_Act. Output Voltage [V]":dbl, "meTEC_CH2_Object Temperature [°C]":dbl, "meTEC_CH2_Sink Temperature [°C]":dbl, "meTEC_CH1_Error Parameter":i32, "meTEC_CH1_Error Instance":i32, "meTEC_CH1_Error No.":i32, "meTEC_CH1_Device Status":T7, "meTEC_CH1_Temperature Stability":T6, "meTEC_CH1_Act. Output Current [A]":dbl, "meTEC_CH1_Act. Output Voltage [V]":dbl, "meTEC_CH1_Object Temperature [°C]":dbl, "meTEC_CH1_Sink Temperature [°C]":dbl}}
  T28 = cluster{"current time":timestamp, "DataOut":cluster{"meTEC_CH2_Temperature Stability":T6, "meTEC_CH2_Act. Output Current [A]":dbl, "meTEC_CH2_Act. Output Voltage [V]":dbl, "meTEC_CH2_Object Temperature [°C]":dbl, "meTEC_CH2_Sink Temperature [°C]":dbl, "meTEC_CH1_Error Parameter":i32, "meTEC_CH1_Error Instance":i32, "meTEC_CH1_Error No.":i32, "meTEC_CH1_Device Status":T7, "meTEC_CH1_Temperature Stability":T6, "meTEC_CH1_Act. Output Current [A]":dbl, "meTEC_CH1_Act. Output Voltage [V]":dbl, "meTEC_CH1_Object Temperature [°C]":dbl, "meTEC_CH1_Sink Temperature [°C]":dbl}}[]
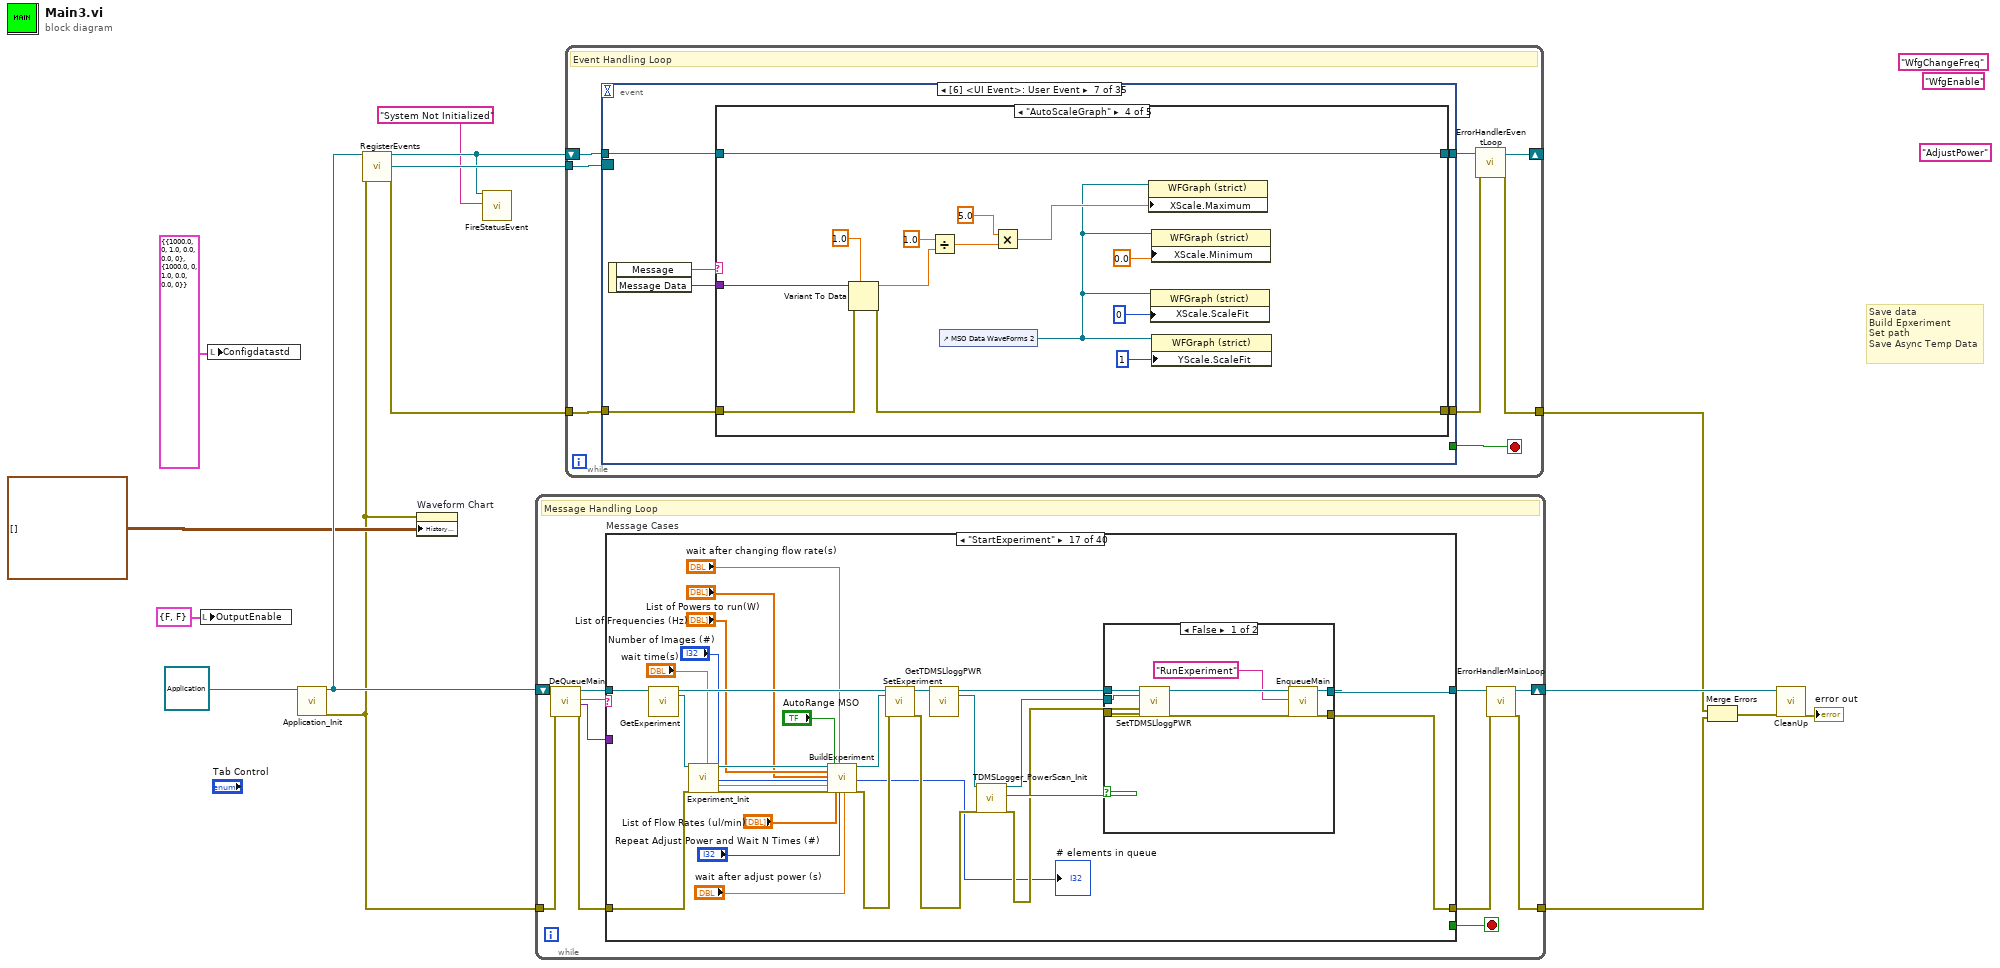
[diagram p0: block diagram]
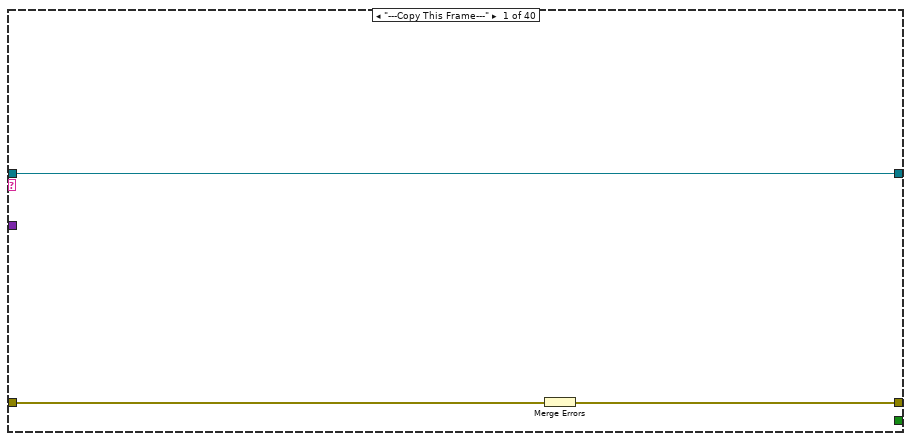
[diagram p2: hidden frame]
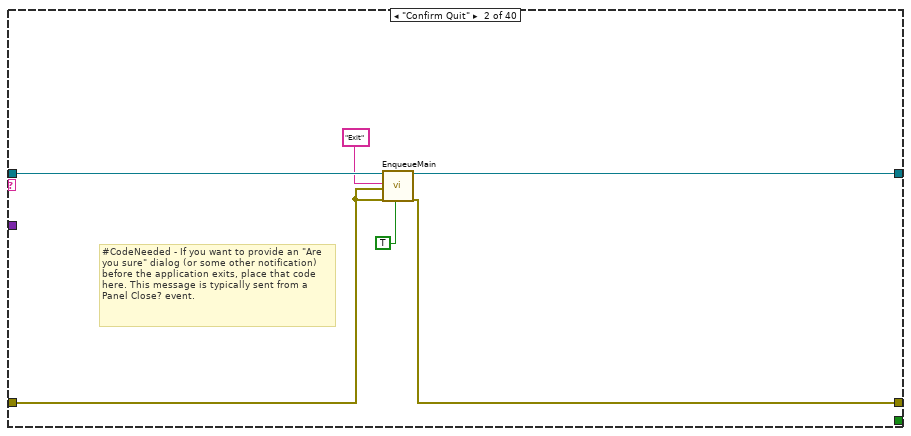
[diagram p3: hidden frame]
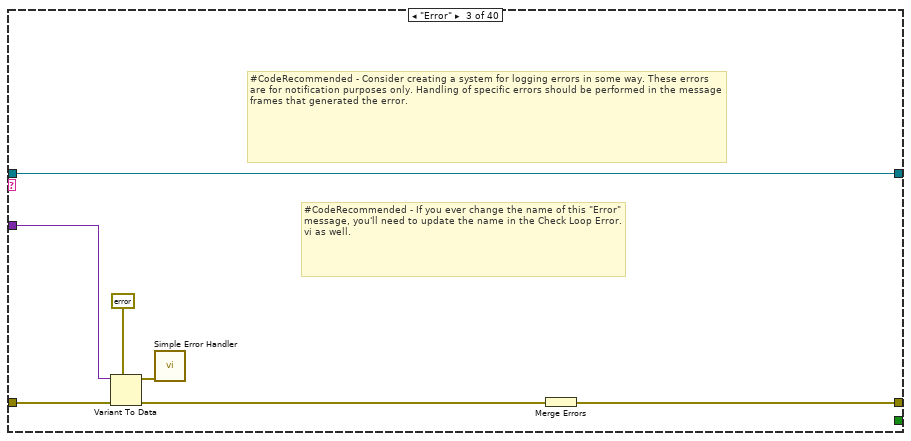
[diagram p4: hidden frame]
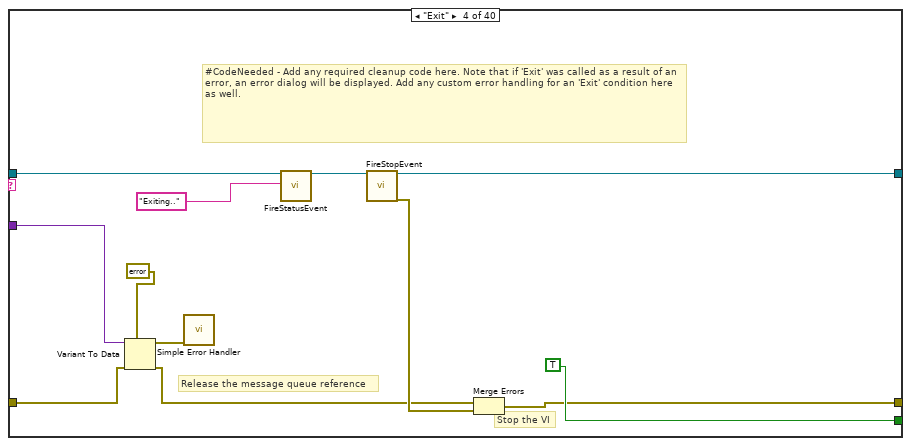
[diagram p5: hidden frame]
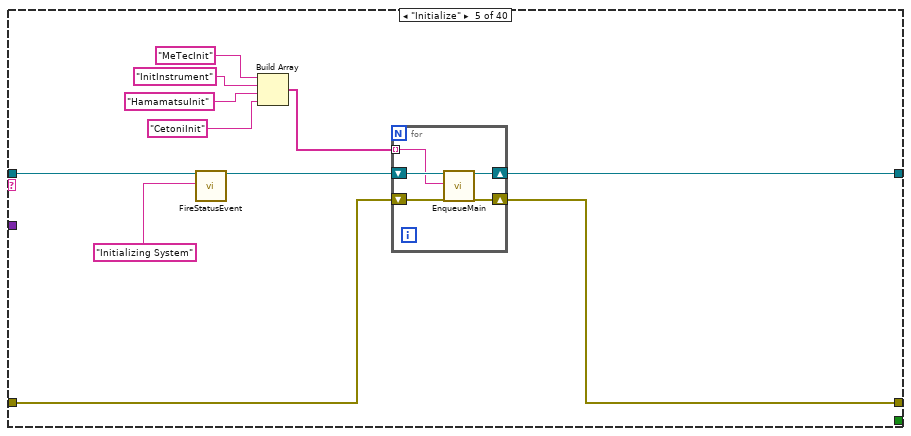
[diagram p6: hidden frame]
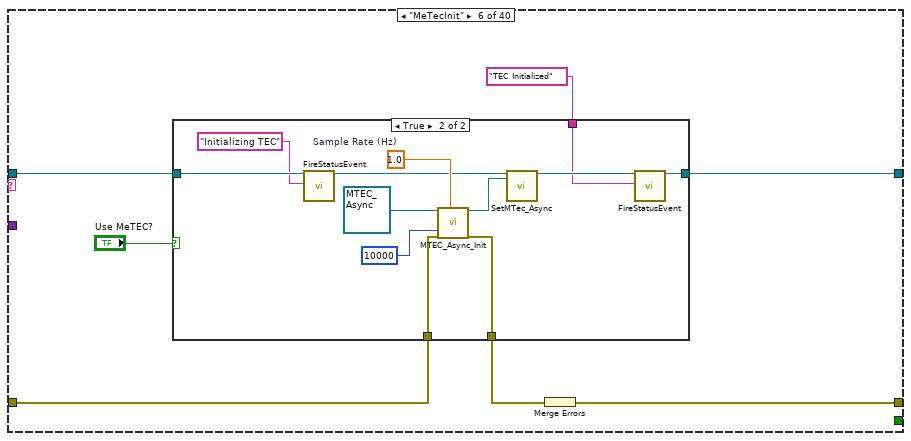
[diagram p7: hidden frame]
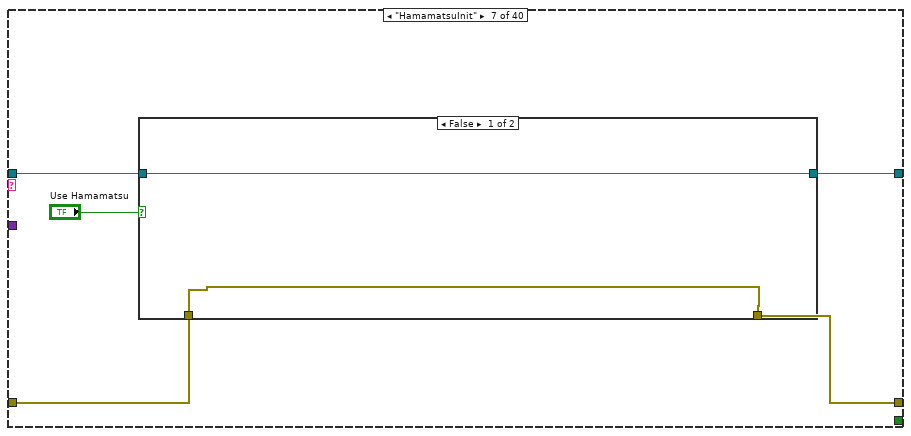
[diagram p9: hidden frame]
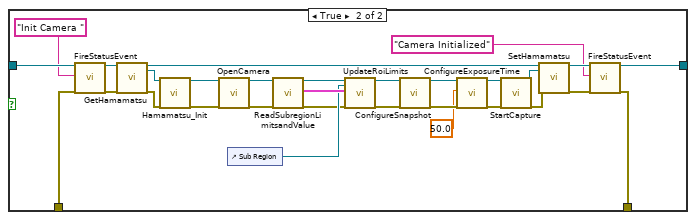
[diagram p10: hidden frame]
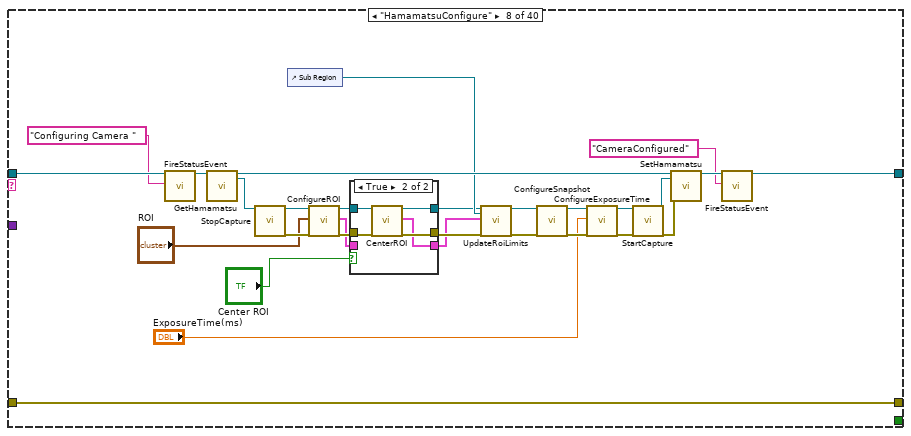
[diagram p11: hidden frame]
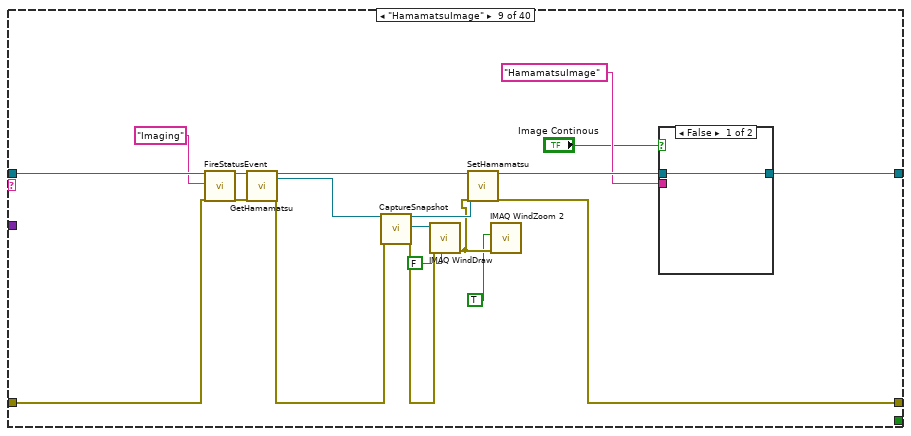
[diagram p13: hidden frame]
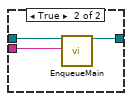
[diagram p14: hidden frame]
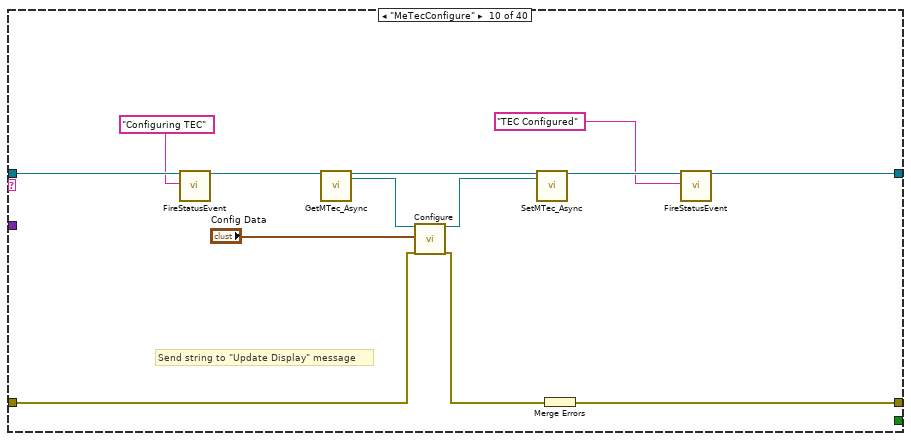
[diagram p15: hidden frame]
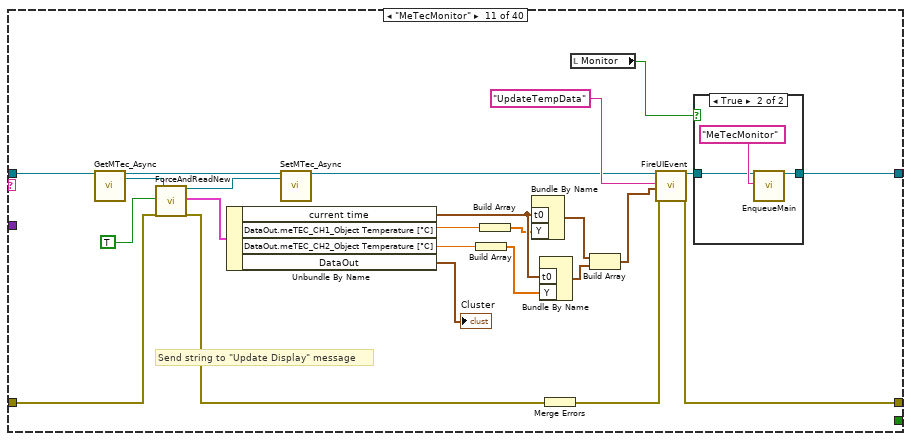
[diagram p16: hidden frame]
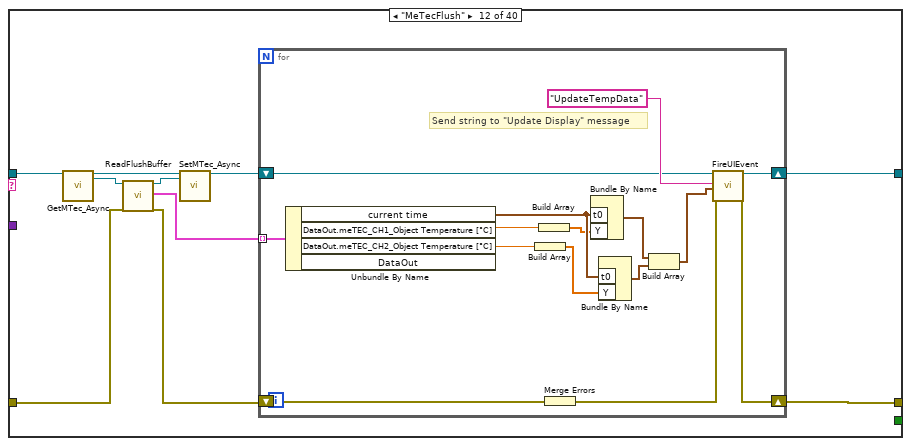
[diagram p18: hidden frame]
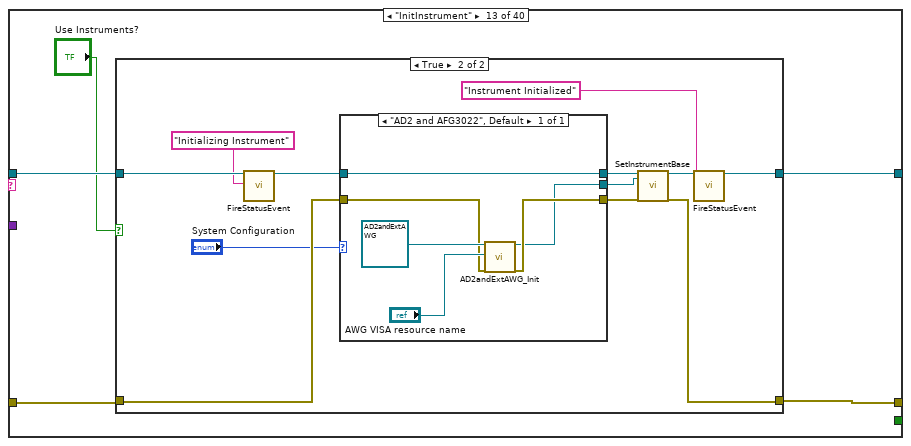
[diagram p19: hidden frame]
diagram:
  (unwired) "AdjustPower" ("Message")
  (unwired) "WfgEnable" ("Message")
  (unwired) "WfgChangeFreq" ("Message")
  # "Save data \nBuild Epxeriment\nSet path\nSave Async Temp Data"
  n1 = local write "OutputEnable"(T13 {"Enable Output WFG Ch1"=FALSE, "Enable Output WFG Ch 2"=FALSE} ("OutputEnable")) -> ()
  n2 = local write "Configdatastd"(T15 {"ConfigDataCh1"={"Frequency Hz (1000 Hz)"=1000.0, "Waveform Function (0: Sine)"=0, "Amplitude (1 Vpp)"=1.0, "DC Offset (0.00 V)"=0.0, "Phase Level (-1)"=0.0, "Phase Unit (0: Radian)"=0}, "ConfigDataCh2"={"Frequency Hz (1000 Hz)"=1000.0, "Waveform Function (0: Sine)"=0, "Amplitude (1 Vpp)"=1.0, "DC Offset (0.00 V)"=0.0, "Phase Level (-1)"=0.0, "Phase Unit (0: Radian)"=0}} ("Configdatastd")) -> ()
  n3 = call "Application_Init.vi"("object in"=refnum<class "Application.lvclass"> refnum ("Application")) -> ("object out"=w12:refnum<class "Application.lvclass">, "error out"=w1:errorcluster)  [unwired: 17 in]
  n4 = call-dynamic "RegisterEvents.vi"("object in"=w12, "error in (no error)"=w1) -> ("object out"=w4:refnum<class "Application.lvclass">, "Event Registration Refnum"=w14:refnum<event-registration>, "error out"=w13:errorcluster)  [unwired: 15 in]
  n5 = property on="Waveform Chart" class="WFChart (strict)"(error in=w1, "History Data"=waveform(dbl)[][] []) -> ()  [unwired: 1 in, 2 out]
  n6 = call-dynamic "FireStatusEvent.vi"("object in"=w4, "Status"="System Not Initialized") -> ()  [unwired: 16 in, 2 out]
  n7 = while {
    tunnel: w1 -> [w16]
    tunnel: [w20] -> w10
    shift-right: [w19] -> w11
    shift-left: w12 -> [w25]
    stop <- w26 stop-if-true
    # "Message Handling Loop"
    n8 = call-dynamic "DeQueueMain.vi"("object in"=w25, "error in (no error)"=w16) -> ("object out"=w24:refnum<class "Application.lvclass">, "Message"=w23:string, "Message Data"=w22:variant, "error out"=w17:errorcluster)  [unwired: 14 in]
    n9 = case "Message Cases" shown="\"StartExperiment\"" w23 {
      selector: w23 -> [_ _ _ _ _ _ _ _ _ _ _ _ _ _ _ _ _ _ _ _ _ _ _ _ _ _ _ _ _ _ _ _ _ _ _ _ _ _ _ w706]
      tunnel: w17 -> [w29 w30 w42 w45 w63 w75 w92 w157 w173 w193 w206 w235 w258 w298 w306 w313 w339 w376 w412 w449 w459 w468 w473 w496 w509 w522 w531 w543 w556 w562 w597 w616 w622 w633 w647 w661 w675 w695 w702 _]
      tunnel: [w28 w35 w37 w53 w64 w77 w93 w157 w175 w201 w223 w239 w257 w280 w305 w311 w344 w380 w409 w450 w458 w469 w482 w499 w510 w523 w532 w544 w557 w563 w598 w617 w628 w641 w654 w666 w670 w683 w701 w707] -> w21
      tunnel: [_ _ _ TRUE _ _ _ _ _ _ _ _ _ _ _ _ _ _ _ _ _ _ _ _ _ _ _ _ _ _ _ _ _ _ _ _ _ _ _ _] -> w26
      tunnel: w22 -> [_ _ w41 w50 _ _ _ _ _ _ _ _ _ _ _ _ _ _ _ _ _ _ w477 w498 _ _ _ _ _ _ w592 w615 w624 w635 w649 w660 _ _ _ _]
      tunnel: w24 -> [w27 w32 w36 w48 w58 w73 w96 w156 w184 w199 w220 w236 w259 w302 w307 w318 w333 w379 w422 w454 w461 w471 w484 w501 w512 w525 w534 w546 w559 w565 w600 w619 w631 w644 w657 w669 w682 w700 w704 w705]
      tunnel: [w27 w33 w36 w49 w65 w71 w95 w155 w171 w197 w203 w232 w256 w284 w304 w321 w348 w381 w421 w452 w460 w470 w483 w500 w511 w515 w533 w538 w558 w564 w596 w618 w621 w642 w655 w659 w674 w694 w703 w705] -> w18
      frame "---Copy This Frame---" {
        # "Duplicate this frame when creating new messages.  Change this comment in the duplicated frame to describe this message."
        n10 = Merge Errors(w29) -> (w28:errorcluster)
      }
      frame "Confirm Quit" {
        # "#CodeNeeded - If you want to provide an \"Are you sure\" dialog (or some other notification) before the application exits, place that code here. This message is typically sent from a Panel Close? event."
        # "Confirm Quit - Message that can confirm whether or not the user wants to exit the application."
        n11 = call-dynamic "EnqueueMain.vi"("object in"=w32, "Message"="Exit", "Message Data"=w30, "error in (no error)"=w30, "Priority Message? (F)"=TRUE) -> ("object out"=w33:refnum<class "Application.lvclass">, "error out"=w35:errorcluster)  [unwired: 13 in]
      }
      frame "Error" {
        # "#CodeRecommended - If you ever change the name of this \"Error\" message, you'll need to update the name in the Check Loop Error.vi as well."
        # "#CodeRecommended - Consider creating a system for logging errors in some way. These errors are for notification purposes only. Handling of specific errors should be performed in the message frames that generated the error."
        # "Error - Display an error dialog. This message is sent by the \"Error Handler\" VIs at the end of other loops in this application."
        n12 = Variant To Data(error in=w42, type=errorcluster {"status"=FALSE, "code"=0, "source"=""} ("error constant"), Variant=w41) -> (data=w39:errorcluster, error out=w38:errorcluster)
        n13 = call <vilib>:"Simple Error Handler.vi"("error in (no error)"=w39) -> ()  [unwired: 4 in, 5 out]
        n14 = Merge Errors(w38) -> (w37:errorcluster)
      }
      frame "Exit" {
        # "Stop the VI"
        # "Release the message queue reference"
        # "#CodeNeeded - Add any required cleanup code here. Note that if 'Exit' was called as a result of an error, an error dialog will be displayed. Add any custom error handling for an 'Exit' condition here as well."
        # "Exit - Exit the application."
        n15 = Variant To Data(error in=w45, type=errorcluster {"status"=FALSE, "code"=0, "source"=""} ("error constant"), Variant=w50) -> (data=w51:errorcluster, error out=w46:errorcluster)
        n16 = call <vilib>:"Simple Error Handler.vi"("error in (no error)"=w51) -> ()  [unwired: 4 in, 5 out]
        n17 = call-dynamic "FireStatusEvent.vi"("object in"=w48, "Status"="Exiting..") -> ("object out"=w44:refnum<class "Application.lvclass">)  [unwired: 16 in, 1 out]
        n18 = call-dynamic "FireStopEvent.vi"("object in"=w44) -> ("object out"=w49:refnum<class "Application.lvclass">, "error out"=w47:errorcluster)  [unwired: 17 in]
        n19 = Merge Errors(w46, w47) -> (w53:errorcluster)
      }
      frame "Initialize" {
        # "Initialize - All initialization work should take place in this message, since other loops can potentially enqueue messages that execute immediately after this one."
        n20 = call-dynamic "FireStatusEvent.vi"("object in"=w58, "Status"="Initializing System") -> ("object out"=w59:refnum<class "Application.lvclass">)  [unwired: 16 in, 1 out]
        n21 = Build Array("MeTecInit" ("Message"), "InitInstrument" ("Message"), "HamamatsuInit" ("Message"), "CetoniInit" ("Message")) -> (w62:string[])
        n22 = for {
          shift-right: [w70] -> w65
          shift-left: w59 -> [w69]
          shift-right: [w68] -> w64
          shift-left: w63 -> [w67]
          tunnel: w62 -> [w66] mode=indexing
          n23 = call-dynamic "EnqueueMain.vi"("object in"=w69, "Message"=w66, "error in (no error)"=w67) -> ("object out"=w70:refnum<class "Application.lvclass">, "error out"=w68:errorcluster)  [unwired: 15 in]
        }
      }
      frame "MeTecInit" {
        # "Something - Replace this message with functionality for your own application."
        n24 = case shown="True" "Use MeTEC?" {
          tunnel: [w79 w90] -> w76
          tunnel: w75 -> [w79 w91]
          tunnel: w73 -> [w78 w85]
          tunnel: "TEC Initialized" ("Status") -> [_ w81]
          tunnel: [w78 w80] -> w71
          frame False {
          }
          frame True {
            w88 = 1.0  # Sample Rate (Hz)
            n25 = call-dynamic "FireStatusEvent.vi"("object in"=w85, "Status"="Initializing TEC") -> ("object out"=w83:refnum<class "Application.lvclass">)  [unwired: 16 in, 1 out]
            n26 = call "MTEC_Async_Init.vi"("object in"=refnum<class "MTEC_Async.lvclass"> refnum, "SW Buffer Size"=10000, "error in (no error)"=w91, "Sample Rate (Hz)"=w88) -> ("object out"=w87:refnum<class "MTEC_Async.lvclass">, "error out"=w90:errorcluster)  [unwired: 14 in]
            n27 = call-dynamic "SetMTec_Async.vi"("object in"=w83, "MTec_Async"=w87) -> ("object out"=w82:refnum<class "Application.lvclass">)  [unwired: 16 in, 1 out]
            n28 = call-dynamic "FireStatusEvent.vi"("object in"=w82, "Status"=w81) -> ("object out"=w80:refnum<class "Application.lvclass">)  [unwired: 16 in, 1 out]
          }
        }
        n29 = Merge Errors(w76) -> (w77:errorcluster)
      }
      frame "HamamatsuInit" {
        n30 = case shown="False" "Use Hamamatsu" {
          tunnel: w96 -> [w98 w128]
          tunnel: [w98 w121] -> w95
          tunnel: [w97 w102] -> w93
          tunnel: w92 -> [w97 w101]
          frame False {
          }
          frame True {
            n31 = call-dynamic "FireStatusEvent.vi"("object in"=w128, "Status"="Init Camera ", "error in (no error)"=w101) -> ("object out"=w123:refnum<class "Application.lvclass">, "error out"=w100:errorcluster)  [unwired: 15 in]
            n32 = call-dynamic "GetHamamatsu.vi"("object in"=w123, "error in (no error)"=w100) -> ("object out"=w127:refnum<class "Application.lvclass">, "Hamamatsu"=w126:refnum<class "Hamamatsu.lvclass">, "error out"=w99:errorcluster)  [unwired: 15 in]
            n33 = call "Hamamatsu_Init.vi"("object in"=w126, "error in (no error)"=w99) -> ("object out"=w125:refnum<class "Hamamatsu.lvclass">, "error out"=w119:errorcluster)  [unwired: 16 in]
            n34 = call-dynamic "OpenCamera.vi"("object in"=w125, "error in (no error)"=w119) -> ("object out"=w111:refnum<class "Hamamatsu.lvclass">, "error out"=w105:errorcluster)  [unwired: 15 in, 1 out]
            n35 = control-ref of="Sub Region"() -> (w109:refnum<vi>)
            n36 = call-dynamic "ReadSubregionLimitsandValue.vi"("object in"=w111, "error in (no error)"=w105) -> ("object out"=w108:refnum<class "Hamamatsu.lvclass">, "Sub Region"=w110:T24, "error out"=w104:errorcluster)  [unwired: 15 in]
            n37 = call-dynamic "UpdateRoiLimits.vi"("object in"=w108, "reference to front panel item"=w109, "SubRegionLimits"=w110, "error in (no error)"=w104) -> ("object out"=w107:refnum<class "Hamamatsu.lvclass">, "error out"=w106:errorcluster)  [unwired: 14 in]
            n38 = call-dynamic "ConfigureSnapshot.vi"("object in"=w107, "error in (no error)"=w106) -> ("object out"=w117:refnum<class "Hamamatsu.lvclass">, "error out"=w118:errorcluster)  [unwired: 16 in]
            n39 = call-dynamic "ConfigureExposureTime.vi"("object in"=w117, "ExposureTime(ms)"=50.0, "error in (no error)"=w118) -> ("object out"=w115:refnum<class "Hamamatsu.lvclass">, "error out"=w114:errorcluster)  [unwired: 15 in]
            n40 = call-dynamic "StartCapture.vi"("object in"=w115, "error in (no error)"=w114) -> ("object out"=w113:refnum<class "Hamamatsu.lvclass">, "error out"=w112:errorcluster)  [unwired: 16 in]
            n41 = call-dynamic "SetHamamatsu.vi"("object in"=w127, "Hamamatsu"=w113, "error in (no error)"=w112) -> ("object out"=w124:refnum<class "Application.lvclass">, "error out"=w103:errorcluster)  [unwired: 15 in]
            n42 = call-dynamic "FireStatusEvent.vi"("object in"=w124, "Status"="Camera Initialized", "error in (no error)"=w103) -> ("object out"=w121:refnum<class "Application.lvclass">, "error out"=w102:errorcluster)  [unwired: 15 in]
          }
        }
      }
      frame "HamamatsuConfigure" {
        n43 = call-dynamic "FireStatusEvent.vi"("object in"=w156, "Status"="Configuring Camera ") -> ("object out"=w152:refnum<class "Application.lvclass">)  [unwired: 16 in, 1 out]
        n44 = call-dynamic "GetHamamatsu.vi"("object in"=w152) -> ("object out"=w154:refnum<class "Application.lvclass">, "Hamamatsu"=w142:refnum<class "Hamamatsu.lvclass">)  [unwired: 16 in, 1 out]
        n45 = call-dynamic "StopCapture.vi"("object in"=w142) -> ("object out"=w141:refnum<class "Hamamatsu.lvclass">, "error out"=w140:errorcluster)  [unwired: 17 in]
        n46 = control-ref of="Sub Region"() -> (w136:refnum<vi>)
        n47 = call-dynamic "ConfigureROI.vi"("object in"=w141, "Sub Region"="ROI", "error in (no error)"=w140) -> ("object out"=w138:refnum<class "Hamamatsu.lvclass">, "SubRegionLimits"=w135:T25, "error out"=w137:errorcluster)  [unwired: 14 in]
        n48 = case shown="True" "Center ROI" {
          tunnel: w138 -> [w158 w165]
          tunnel: [w158 w164] -> w134
          tunnel: w137 -> [w159 w163]
          tunnel: [w159 w162] -> w132
          tunnel: w135 -> [w160 _]
          tunnel: [w160 w161] -> w130
          frame False {
          }
          frame True {
            n49 = call-dynamic "CenterROI.vi"("object in"=w165, "error in (no error)"=w163) -> ("object out"=w164:refnum<class "Hamamatsu.lvclass">, "Sub Region"=w161:T24, "error out"=w162:errorcluster)  [unwired: 15 in]
          }
        }
        n50 = call-dynamic "UpdateRoiLimits.vi"("object in"=w134, "reference to front panel item"=w136, "SubRegionLimits"=w130, "error in (no error)"=w132) -> ("object out"=w133:refnum<class "Hamamatsu.lvclass">, "error out"=w131:errorcluster)  [unwired: 14 in]
        n51 = call-dynamic "ConfigureSnapshot.vi"("object in"=w133, "error in (no error)"=w131) -> ("object out"=w148:refnum<class "Hamamatsu.lvclass">, "error out"=w149:errorcluster)  [unwired: 16 in]
        n52 = call-dynamic "ConfigureExposureTime.vi"("object in"=w148, "ExposureTime(ms)"="ExposureTime(ms)", "error in (no error)"=w149) -> ("object out"=w146:refnum<class "Hamamatsu.lvclass">, "error out"=w145:errorcluster)  [unwired: 15 in]
        n53 = call-dynamic "StartCapture.vi"("object in"=w146, "error in (no error)"=w145) -> ("object out"=w144:refnum<class "Hamamatsu.lvclass">, "error out"=w143:errorcluster)  [unwired: 16 in]
        n54 = call-dynamic "SetHamamatsu.vi"("object in"=w154, "Hamamatsu"=w144, "error in (no error)"=w143) -> ("object out"=w153:refnum<class "Application.lvclass">)  [unwired: 15 in, 1 out]
        n55 = call-dynamic "FireStatusEvent.vi"("object in"=w153, "Status"="CameraConfigured") -> ("object out"=w155:refnum<class "Application.lvclass">)  [unwired: 16 in, 1 out]
      }
      frame "HamamatsuImage" {
        n56 = call-dynamic "FireStatusEvent.vi"("object in"=w184, "Status"="Imaging", "error in (no error)"=w173) -> ("object out"=w181:refnum<class "Application.lvclass">, "error out"=w174:errorcluster)  [unwired: 15 in]
        n57 = call-dynamic "GetHamamatsu.vi"("object in"=w181, "error in (no error)"=w174) -> ("object out"=w183:refnum<class "Application.lvclass">, "Hamamatsu"=w179:refnum<class "Hamamatsu.lvclass">, "error out"=w172:errorcluster)  [unwired: 15 in]
        n58 = call-dynamic "CaptureSnapshot.vi"("object in"=w179, "error in (no error)"=w172) -> ("object out"=w178:refnum<class "Hamamatsu.lvclass">, "FreeRunningImage"=w177:T26, "error out"=w176:errorcluster)  [unwired: 14 in, 1 out]
        n59 = call "IMAQ WindDraw"("Resize to Image Size? (Y)"=FALSE, "error in (no error)"=w176, "Image"=w177) -> ("error out"=w167:errorcluster)  [unwired: 7 in, 1 out]
        n60 = call-dynamic "SetHamamatsu.vi"("object in"=w183, "Hamamatsu"=w178, "error in (no error)"=w167) -> ("object out"=w182:refnum<class "Application.lvclass">, "error out"=w175:errorcluster)  [unwired: 15 in]
        n61 = call "IMAQ WindZoom 2"("error in (no error)"=w167, "Zoom to Fit? (False)"=TRUE) -> ()  [unwired: 6 in, 4 out]
        n62 = case shown="False" "Image Continous" {
          tunnel: w182 -> [w185 w188]
          tunnel: [w185 w187] -> w171
          tunnel: "HamamatsuImage" ("Message") -> [_ w186]
          frame False {
          }
          frame True {
            n63 = call-dynamic "EnqueueMain.vi"("object in"=w188, "Message"=w186) -> ("object out"=w187:refnum<class "Application.lvclass">)  [unwired: 16 in, 1 out]
          }
        }
      }
      frame "MeTecConfigure" {
        # "Send string to \"Update Display\" message"
        # "Something - Replace this message with functionality for your own application."
        n64 = call-dynamic "FireStatusEvent.vi"("object in"=w199, "Status"="Configuring TEC") -> ("object out"=w195:refnum<class "Application.lvclass">)  [unwired: 16 in, 1 out]
        n65 = call-dynamic "GetMTec_Async.vi"("object in"=w195) -> ("object out"=w198:refnum<class "Application.lvclass">, "MTec_Async"=w191:refnum<class "MTEC_Async.lvclass">)  [unwired: 16 in, 1 out]
        n66 = call-dynamic "Configure.vi"("object in"=w191, "Config Data"="Config Data", "error in (no error)"=w193) -> ("object out"=w190:refnum<class "MTEC_Async.lvclass">, "error out"=w192:errorcluster)  [unwired: 15 in]
        n67 = call-dynamic "SetMTec_Async.vi"("object in"=w198, "MTec_Async"=w190) -> ("object out"=w200:refnum<class "Application.lvclass">)  [unwired: 16 in, 1 out]
        n68 = Merge Errors(w192) -> (w201:errorcluster)
        n69 = call-dynamic "FireStatusEvent.vi"("object in"=w200, "Status"="TEC Configured") -> ("object out"=w197:refnum<class "Application.lvclass">)  [unwired: 16 in, 1 out]
      }
      frame "MeTecMonitor" {
        # "Send string to \"Update Display\" message"
        # "Something - Replace this message with functionality for your own application."
        n70 = call-dynamic "GetMTec_Async.vi"("object in"=w220) -> ("object out"=w221:refnum<class "Application.lvclass">, "MTec_Async"=w210:refnum<class "MTEC_Async.lvclass">)  [unwired: 16 in, 1 out]
        n71 = call-dynamic "ForceAndReadNew.vi"("object in"=w210, "Buffer Values"=TRUE, "error in (no error)"=w206) -> ("object out"=w209:refnum<class "MTEC_Async.lvclass">, "Cluster"=w208:T27, "error out"=w207:errorcluster)  [unwired: 14 in]
        n72 = Unbundle By Name(w208) -> ("current time"=w215:timestamp, "DataOut.meTEC_CH1_Object Temperature [°C]"=w219:dbl, "DataOut.meTEC_CH2_Object Temperature [°C]"=w212:dbl, "DataOut"=→"Cluster":T8)
        n73 = call-dynamic "SetMTec_Async.vi"("object in"=w221, "MTec_Async"=w209) -> ("object out"=w222:refnum<class "Application.lvclass">)  [unwired: 16 in, 1 out]
        n74 = Build Array(w212) -> (w211:dbl[])
        n75 = Build Array(w219) -> (w214:dbl[])
        n76 = Bundle By Name("t0"=w215, "Y"=w214) -> (w217:waveform(dbl))  [unwired: 1 in]
        n77 = Bundle By Name("t0"=w215, "Y"=w211) -> (w216:waveform(dbl))  [unwired: 1 in]
        n78 = Merge Errors(w207) -> (w224:errorcluster)
        n79 = local read "Monitor"() -> (w202:bool)
        n80 = Build Array(w217, w216) -> (w213:waveform(dbl)[])
        n81 = call-dynamic "FireUIEvent.vi"("object in"=w222, "Message"="UpdateTempData", "Message Data"=w213, "error in (no error)"=w224) -> ("object out"=w204:refnum<class "Application.lvclass">, "error out"=w223:errorcluster)  [unwired: 14 in]
        n82 = case shown="True" w202 {
          tunnel: w204 -> [w226 w228]
          tunnel: [w226 w227] -> w203
          frame False {
          }
          frame True {
            n83 = call-dynamic "EnqueueMain.vi"("object in"=w228, "Message"="MeTecMonitor") -> ("object out"=w227:refnum<class "Application.lvclass">)  [unwired: 16 in, 1 out]
          }
        }
      }
      frame "MeTecFlush" {
        # "Something - Replace this message with functionality for your own application."
        n84 = call-dynamic "GetMTec_Async.vi"("object in"=w236) -> ("object out"=w237:refnum<class "Application.lvclass">, "MTec_Async"=w233:refnum<class "MTEC_Async.lvclass">)  [unwired: 16 in, 1 out]
        n85 = call-dynamic "ReadFlushBuffer.vi"("object in"=w233, "error in (no error)"=w235) -> ("object out"=w231:refnum<class "MTEC_Async.lvclass">, "Stored Data"=w230:T28, "error out"=w234:errorcluster)  [unwired: 15 in]
        n86 = call-dynamic "SetMTec_Async.vi"("object in"=w237, "MTec_Async"=w231) -> ("object out"=w238:refnum<class "Application.lvclass">)  [unwired: 16 in, 1 out]
        n87 = for {
          tunnel: w230 -> [w240] mode=indexing
          shift-right: [w241] -> w232
          shift-left: w238 -> [w251]
          shift-right: [w252] -> w239
          shift-left: w234 -> [w242]
          # "Send string to \"Update Display\" message"
          n88 = Unbundle By Name(w240) -> ("current time"=w247:timestamp, "DataOut.meTEC_CH1_Object Temperature [°C]"=w250:dbl, "DataOut.meTEC_CH2_Object Temperature [°C]"=w244:dbl)  [unwired: 1 out]
          n89 = Build Array(w244) -> (w243:dbl[])
          n90 = Build Array(w250) -> (w246:dbl[])
          n91 = Merge Errors(w242) -> (w253:errorcluster)
          n92 = Bundle By Name("t0"=w247, "Y"=w246) -> (w249:waveform(dbl))  [unwired: 1 in]
          n93 = Bundle By Name("t0"=w247, "Y"=w243) -> (w248:waveform(dbl))  [unwired: 1 in]
          n94 = Build Array(w249, w248) -> (w245:waveform(dbl)[])
          n95 = call-dynamic "FireUIEvent.vi"("object in"=w251, "Message"="UpdateTempData", "Message Data"=w245, "error in (no error)"=w253) -> ("object out"=w241:refnum<class "Application.lvclass">, "error out"=w252:errorcluster)  [unwired: 14 in]
        }
      }
      frame "InitInstrument" {
        n96 = case shown="True" "Use Instruments?" {
          tunnel: w259 -> [w261 w273]
          tunnel: w258 -> [w260 w272]
          tunnel: [w260 w268] -> w257
          tunnel: [w261 w263] -> w256
          frame False {
          }
          frame True {
            n97 = call-dynamic "FireStatusEvent.vi"("object in"=w273, "Status"="Initializing Instrument") -> ("object out"=w265:refnum<class "Application.lvclass">)  [unwired: 16 in, 1 out]
            n98 = case shown="\"AD2 and AFG3022\", Default" "System Configuration" {
              tunnel: w265 -> [w275]
              tunnel: w272 -> [w277]
              tunnel: [w276] -> w270
              tunnel: [w275] -> w267
              tunnel: [w274] -> w266
              frame "AD2 and AFG3022", Default {
                n99 = call "AD2andExtAWG_Init.vi"("object in"=refnum<class "AD2andExtAWG.lvclass"> refnum ("AD2andExtAWG"), "VISA resource name"="AWG VISA resource name", "error in (no error)"=w277) -> ("object out"=w274:refnum<class "AD2andExtAWG.lvclass">, "error out"=w276:errorcluster)  [unwired: 15 in]
              }
            }
            n100 = call-dynamic "SetInstrumentBase.vi"("object in"=w267, "InstrumentBase"=w266, "error in (no error)"=w270) -> ("object out"=w269:refnum<class "Application.lvclass">, "error out"=w268:errorcluster)  [unwired: 15 in]
            n101 = call-dynamic "FireStatusEvent.vi"("object in"=w269, "Status"="Instrument Initialized") -> ("object out"=w263:refnum<class "Application.lvclass">)  [unwired: 16 in, 1 out]
          }
        }
      }
      frame "MeTecReset" {
        n102 = call-dynamic "FireStatusEvent.vi"("object in"=w302, "Status"="Reseting Tec ") -> ("object out"=w296:refnum<class "Application.lvclass">)  [unwired: 16 in, 1 out]
        n103 = call-dynamic "GetMTec.vi"("object in"=w296, "error in (no error)"=w298) -> ("object out"=w301:refnum<class "Application.lvclass">, "MTec"=w299:refnum<class "MTec.lvclass">, "error out"=w297:errorcluster)  [unwired: 15 in]
        n104 = call-dynamic "Reset.vi"("object in"=w299, "error in (no error)"=w297) -> ("object out"=w295:refnum<class "MTec.lvclass">, "error out"=w287:errorcluster)  [unwired: 16 in]
        n105 = call-dynamic "FireStatusEvent.vi"("object in"=w301, "Status"="Closing Tec Connection", "error in (no error)"=w287) -> ("object out"=w292:refnum<class "Application.lvclass">, "error out"=w286:errorcluster)  [unwired: 15 in]
        n106 = call-dynamic "CleanUp.vi"("object in"=w295, "error in (no error)"=w286) -> ("object out"=w294:refnum<class "MTec.lvclass">, "error out"=w288:errorcluster)  [unwired: 16 in]
        n107 = call-dynamic "FireStatusEvent.vi"("object in"=w292, "Status"="Reestablishing Tec Connection", "error in (no error)"=w288) -> ("object out"=w291:refnum<class "Application.lvclass">, "error out"=w290:errorcluster)  [unwired: 15 in]
        n108 = call "MTec_Init.vi"("object in"=w294, "error in (no error)"=w290) -> ("object out"=w293:refnum<class "MTec.lvclass">, "error out"=w289:errorcluster)  [unwired: 16 in]
        n109 = call-dynamic "SetMTec.vi"("object in"=w291, "MTec"=w293, "error in (no error)"=w289) -> ("object out"=w300:refnum<class "Application.lvclass">, "error out"=w280:errorcluster)  [unwired: 15 in]
        n110 = call-dynamic "FireStatusEvent.vi"("object in"=w300, "Status"="Tec Reset!", "error in (no error)"=w280) -> ("object out"=w284:refnum<class "Application.lvclass">)  [unwired: 15 in, 1 out]
      }
      frame "Abort" {
        # "Might have to close fileref here etc.."
        n111 = call-dynamic "FlushMainQueue.vi"("object in"=w307, "error in (no error)"=w306) -> ("object out"=w308:refnum<class "Application.lvclass">, "error out"=w305:errorcluster)  [unwired: 15 in, 1 out]
        n112 = call-dynamic "FireStatusEvent.vi"("object in"=w308, "Status"="Sequence Aborted") -> ("object out"=w304:refnum<class "Application.lvclass">)  [unwired: 16 in, 1 out]
      }
      frame "StartPwrScan" {
        n113 = call-dynamic "GetInstrumentBase.vi"("object in"=w318, "error in (no error)"=w313) -> ("object out"=w320:refnum<class "Application.lvclass">, "InstrumentBase"=w317:refnum<class "InstrumentBase.lvclass">, "error out"=w314:errorcluster)  [unwired: 15 in]
        n114 = call-dynamic "StartPowerScan.vi"("object in"=w317, "PwrScanSettings"="PwrScanSettings", "CurrentProbeScaling(V/A)"="CurrentProbeScaling(V/A)", "error in (no error)"=w314) -> ("object out"=w316:refnum<class "InstrumentBase.lvclass">, "error out"=w312:errorcluster)  [unwired: 14 in]
        n115 = call-dynamic "SetInstrumentBase.vi"("object in"=w320, "InstrumentBase"=w316, "error in (no error)"=w312) -> ("object out"=w319:refnum<class "Application.lvclass">, "error out"=w311:errorcluster)  [unwired: 15 in]
        n116 = call-dynamic "EnqueueMain.vi"("object in"=w319, "Message"="RunPwrScan") -> ("object out"=w321:refnum<class "Application.lvclass">)  [unwired: 16 in, 1 out]
      }
      frame "StartExperiment" {
        n117 = call-dynamic "GetExperiment.vi"("object in"=w333) -> ("object out"=w334:refnum<class "Application.lvclass">, "Experiment"=w332:refnum<class "Experiment.lvclass">)  [unwired: 16 in, 1 out]
        n118 = call "Experiment_Init.vi"("object in"=w332, "error in (no error)"=w339) -> ("object out"=w341:refnum<class "Experiment.lvclass">, "error out"=w340:errorcluster)  [unwired: 16 in]
        n119 = call-dynamic "BuildExperiment.vi"("object in"=w341, "List of Frequencies"="List of Frequencies (Hz)", "List of Powers to run(W)"="List of Powers to run(W)", "Number of Images"="Number of Images (#)", "wait time(s)"="wait time(s)", "error in (no error)"=w340, "AutoRange MSO"="AutoRange MSO", "Flow"="List of Flow Rates (ul/min)", "wait after changing flow rate(s)"="wait after changing flow rate(s)", "Repeat Adjust Power and Wait N Times"="Repeat Adjust Power and Wait N Times (#)", "wait after adjust power"="wait after adjust power (s)") -> ("object out"=w337:refnum<class "Experiment.lvclass">, "# elements in queue"=→"# elements in queue":i32, "error out"=w336:errorcluster)  [unwired: 6 in]
        n120 = call-dynamic "SetExperiment.vi"("object in"=w334, "Experiment"=w337, "error in (no error)"=w336) -> ("object out"=w338:refnum<class "Application.lvclass">, "error out"=w335:errorcluster)  [unwired: 15 in]
        n121 = call-dynamic "GetTDMSLloggPWR.vi"("object in"=w338) -> ("object out"=w346:refnum<class "Application.lvclass">, "TDMSLloggPWR"=w347:refnum<class "TDMSLogger_PowerScan.lvclass">)  [unwired: 16 in, 1 out]
        n122 = call "TDMSLogger_PowerScan_Init.vi"("object in"=w347, "error in (no error)"=w335) -> ("object out"=w342:refnum<class "TDMSLogger_PowerScan.lvclass">, "cancelled"=w345:bool, "error out"=w343:errorcluster)  [unwired: 15 in]
        n123 = case shown="False" w345 {
          tunnel: [w356 w360] -> w348
          tunnel: w346 -> [w354 w361]
          tunnel: [w352 w358] -> w344
          tunnel: w343 -> [w351 w359]
          tunnel: w342 -> [w350 _]
          frame False {
            n124 = call-dynamic "SetTDMSLloggPWR.vi"("object in"=w354, "TDMSLloggPWR"=w350, "error in (no error)"=w351) -> ("object out"=w355:refnum<class "Application.lvclass">, "error out"=w353:errorcluster)  [unwired: 15 in]
            n125 = call-dynamic "EnqueueMain.vi"("object in"=w355, "Message"="RunExperiment", "error in (no error)"=w353) -> ("object out"=w356:refnum<class "Application.lvclass">, "error out"=w352:errorcluster)  [unwired: 15 in]
          }
          frame True {
            n126 = call-dynamic "FireStatusEvent.vi"("object in"=w361, "Status"="Experiment Complete", "error in (no error)"=w359) -> ("object out"=w360:refnum<class "Application.lvclass">, "error out"=w358:errorcluster)  [unwired: 15 in]
          }
        }
      }
      frame "RunExperiment" {
        n127 = local read "# elements in queue"() -> (w367:i32)
        n128 = call-dynamic "GetExperiment.vi"("object in"=w379) -> ("object out"=w374:refnum<class "Application.lvclass">, "Experiment"=w378:refnum<class "Experiment.lvclass">)  [unwired: 16 in, 1 out]
        n129 = call-dynamic "DequeueExperiment.vi"("object in"=w378, "error in (no error)"=w376) -> ("# elements in queue"=w368:i32, "object out"=w375:refnum<class "Experiment.lvclass">, "Message"=w370:string, "Message Data"=w369:variant, "QueueEmpty"=w377:bool, "error out"=w372:errorcluster)  [unwired: 12 in]
        n130 = call-dynamic "SetExperiment.vi"("object in"=w374, "Experiment"=w375, "error in (no error)"=w372) -> ("object out"=w373:refnum<class "Application.lvclass">, "error out"=w371:errorcluster)  [unwired: 15 in]
        n131 = Divide(x=w368, y=w367) -> (x/y=w366:dbl)
        n132 = Subtract(x=1.0, y=w366) -> (x-y=w364:dbl)
        n133 = Multiply(x=w364, y=100.0) -> (x*y=→"Progress (100%)":dbl)
        n134 = case shown="True" w377 {
          tunnel: [w385 w402] -> w381
          tunnel: w373 -> [w390 w398]
          tunnel: [w382 w395] -> w380
          tunnel: w371 -> [w388 w394]
          tunnel: w370 -> [w389 _]
          tunnel: w369 -> [w387 _]
          frame False {
            n135 = call-dynamic "EnqueueMain.vi"("object in"=w390, "Message"=w389, "Message Data"=w387, "error in (no error)"=w388) -> ("object out"=w391:refnum<class "Application.lvclass">, "error out"=w386:errorcluster)  [unwired: 14 in]
            n136 = call-dynamic "EnqueueMain.vi"("object in"=w391, "Message"="RunExperiment", "error in (no error)"=w386) -> ("object out"=w393:refnum<class "Application.lvclass">, "error out"=w383:errorcluster)  [unwired: 15 in]
            n137 = call-dynamic "FireStatusEvent.vi"("object in"=w393, "Status"="Running Experiment", "error in (no error)"=w383) -> ("object out"=w385:refnum<class "Application.lvclass">, "error out"=w382:errorcluster)  [unwired: 15 in]
          }
          frame True {
            n138 = call-dynamic "GetTDMSLloggPWR.vi"("object in"=w398) -> ("object out"=w400:refnum<class "Application.lvclass">, "TDMSLloggPWR"=w397:refnum<class "TDMSLogger_PowerScan.lvclass">)  [unwired: 16 in, 1 out]
            n139 = call-dynamic "CleanUp.vi"("object in"=w397, "error in (no error)"=w394) -> ("object out"=w396:refnum<class "TDMSLogger_PowerScan.lvclass">, "error out"=w395:errorcluster)  [unwired: 16 in]
            n140 = call-dynamic "SetTDMSLloggPWR.vi"("object in"=w400, "TDMSLloggPWR"=w396) -> ("object out"=w399:refnum<class "Application.lvclass">)  [unwired: 16 in, 1 out]
            n141 = call-dynamic "FireStatusEvent.vi"("object in"=w399, "Status"="Experiment Complete") -> ("object out"=w402:refnum<class "Application.lvclass">)  [unwired: 16 in, 1 out]
          }
        }
      }
      frame "RunPwrScan" {
        n142 = call-dynamic "GetInstrumentBase.vi"("object in"=w422, "error in (no error)"=w412) -> ("object out"=w420:refnum<class "Application.lvclass">, "InstrumentBase"=w418:refnum<class "InstrumentBase.lvclass">, "error out"=w411:errorcluster)  [unwired: 15 in]
        n143 = call-dynamic "RunPowerScan.vi"("object in"=w418, "error in (no error)"=w411) -> ("Impedance"=w404:cluster{dbl[], dbl[]}, "Phase"=w403:cluster{dbl[], dbl[]}, "object out"=w417:refnum<class "InstrumentBase.lvclass">, "PowerScanComplete"=w416:bool, "PowerScanResult"=w406:cluster{"PwrFreq":dbl[], "PwrMeasured":dbl[]}, "Channels array"=w410:waveform(dbl)[], "error out"=w408:errorcluster)  [unwired: 11 in]
        n144 = Unbundle By Name(w406) -> ("PwrMeasured"=w415:dbl[])
        n145 = call-dynamic "SetInstrumentBase.vi"("object in"=w420, "InstrumentBase"=w417, "error in (no error)"=w408) -> ("object out"=w419:refnum<class "Application.lvclass">, "error out"=w407:errorcluster)  [unwired: 15 in]
        n146 = Build Array(w406, w404, w403) -> (→"Power Graph":cluster{"PwrFreq":dbl[], "PwrMeasured":dbl[]}[])
        n147 = Array Max & Min(array=w415) -> (max value=→"max Power":dbl, min value=→"min Power":dbl)  [unwired: 2 out]
        n148 = case shown="False" w416 {
          tunnel: [w434 w438] -> w421
          tunnel: w419 -> [w433 w439]
          tunnel: w410 -> [w430 _]
          tunnel: w407 -> [w427 w435]
          tunnel: [w428 w436] -> w409
          frame False {
            n149 = call-dynamic "FireUIEvent.vi"("object in"=w433, "Message"="UpdateMsoData", "Message Data"=w430, "error in (no error)"=w427) -> ("object out"=w431:refnum<class "Application.lvclass">, "error out"=w425:errorcluster)  [unwired: 14 in]
            n150 = call-dynamic "FireStatusEvent.vi"("object in"=w431, "Status"="Running PowerScan", "error in (no error)"=w425) -> ("object out"=w426:refnum<class "Application.lvclass">, "error out"=w424:errorcluster)  [unwired: 15 in]
            n151 = call-dynamic "EnqueueMain.vi"("object in"=w426, "Message"="RunPwrScan", "error in (no error)"=w424) -> ("object out"=w434:refnum<class "Application.lvclass">, "error out"=w428:errorcluster)  [unwired: 15 in]
          }
          frame True {
            n152 = call-dynamic "FireStatusEvent.vi"("object in"=w439, "Status"="PowerScan Complete", "error in (no error)"=w435) -> ("object out"=w438:refnum<class "Application.lvclass">, "error out"=w436:errorcluster)  [unwired: 15 in]
          }
        }
      }
      frame "MeasurePwr" {
        n153 = local read "CurrentProbeScaling(V/A)"() -> (w445:dbl)
        n154 = call-dynamic "GetInstrumentBase.vi"("object in"=w454, "error in (no error)"=w449) -> ("object out"=w453:refnum<class "Application.lvclass">, "InstrumentBase"=w447:refnum<class "InstrumentBase.lvclass">, "error out"=w444:errorcluster)  [unwired: 15 in]
        n155 = call-dynamic "SetCurrentProbeScaling(VA).vi"("object in"=w447, "CurrentProbeScaling(V/A)"=w445, "error in (no error)"=w444) -> ("object out"=w446:refnum<class "InstrumentBase.lvclass">, "error out"=w443:errorcluster)  [unwired: 15 in]
        n156 = call-dynamic "MeasurePower.vi"("object in"=w446, "error in (no error)"=w443) -> ("impedance (ohm)"=→"impedance (ohm)":dbl, "phase (deg)"=→"phase (deg)":dbl, "object out"=w451:refnum<class "InstrumentBase.lvclass">, "Measured Power"=→"Measured Power":dbl, "error out"=w442:errorcluster)  [unwired: 12 in, 1 out]
        n157 = call-dynamic "SetInstrumentBase.vi"("object in"=w453, "InstrumentBase"=w451, "error in (no error)"=w442) -> ("object out"=w452:refnum<class "Application.lvclass">, "error out"=w450:errorcluster)  [unwired: 15 in]
      }
      frame "CetoniCondRefill" {
        n158 = call-dynamic "ConditionalRefill.vi"("object in"=w461, "Turn Off WFG During Refill"="Turn Off WFG During Refill", "refill below level(uL)"="refill below level(uL)", "refill and \nempty rate(uL/min)"="refill and \nempty rate(uL/min)", "error in (no error)"=w459) -> ("object out"=w460:refnum<class "Application.lvclass">, "error out"=w458:errorcluster)  [unwired: 13 in]
      }
      frame "CetoniRefill" {
        n159 = call-dynamic "GetCetoniPump.vi"("object in"=w471, "error in (no error)"=w468) -> ("object out"=w472:refnum<class "Application.lvclass">, "CetoniPump"=w467:refnum<class "CetoniPump.lvclass">, "error out"=w465:errorcluster)  [unwired: 15 in]
        n160 = local read "refill and \nempty rate(uL/min)"() -> (w462:dbl)
        n161 = local read "index"() -> (w463:i32)
        n162 = call-dynamic "Refill.vi"("object in"=w467, "refill rate"=w462, "index"=w463, "error in (no error)"=w465) -> ("object out"=w466:refnum<class "CetoniPump.lvclass">, "error out"=w464:errorcluster)  [unwired: 14 in]
        n163 = call-dynamic "SetCetoniPump.vi"("object in"=w472, "CetoniPump"=w466, "error in (no error)"=w464) -> ("object out"=w470:refnum<class "Application.lvclass">, "error out"=w469:errorcluster)  [unwired: 15 in]
      }
      frame "CetoniToggleValve" {
        n164 = Variant To Data(error in=w473, type=cluster{"index":i32, "Valve Position":bool} {"index"=0, "Valve Position"=FALSE} ("ValveControl"), Variant=w477) -> (data=w475:cluster{"index":i32, "Valve Position":bool}, error out=w474:errorcluster)
        n165 = call-dynamic "GetCetoniPump.vi"("object in"=w484, "error in (no error)"=w474) -> ("object out"=w485:refnum<class "Application.lvclass">, "CetoniPump"=w481:refnum<class "CetoniPump.lvclass">, "error out"=w479:errorcluster)  [unwired: 15 in]
        n166 = call-dynamic "ToggleValve.vi"("object in"=w481, "ValveControl"=w475, "error in (no error)"=w479) -> ("object out"=w480:refnum<class "CetoniPump.lvclass">, "error out"=w478:errorcluster)  [unwired: 15 in]
        n167 = call-dynamic "SetCetoniPump.vi"("object in"=w485, "CetoniPump"=w480, "error in (no error)"=w478) -> ("object out"=w483:refnum<class "Application.lvclass">, "error out"=w482:errorcluster)  [unwired: 15 in]
      }
      frame "CetoniGoToLevel" {
        n168 = Variant To Data(error in=w496, type=T22 {"index"=0, "Level(ml)"=0.0, "Flow"=0.0} ("GoToLevelSettings"), Variant=w498) -> (data=w490:T22, error out=w497:errorcluster)
        n169 = call-dynamic "GetCetoniPump.vi"("object in"=w501, "error in (no error)"=w497) -> ("object out"=w502:refnum<class "Application.lvclass">, "CetoniPump"=w495:refnum<class "CetoniPump.lvclass">, "error out"=w494:errorcluster)  [unwired: 15 in]
        n170 = call-dynamic "SetFillLevel.vi"("object in"=w495, "GoToLevelSettings"=w490, "error in (no error)"=w494) -> ("object out"=w492:refnum<class "CetoniPump.lvclass">, "Coerced Level"=w488:dbl, "Coerced Flow"=w487:dbl, "error out"=w493:errorcluster)  [unwired: 12 in, 1 out]
        n171 = call-dynamic "SetCetoniPump.vi"("object in"=w502, "CetoniPump"=w492, "error in (no error)"=w493) -> ("object out"=w500:refnum<class "Application.lvclass">, "error out"=w499:errorcluster)  [unwired: 15 in]
        n172 = local read "GoToLevelSettings"() -> (w489:T4)
        n173 = Bundle By Name(cluster=w489, "Level(uL)"=w488, "Flow"=w487) -> (w486:T4)
        n174 = local write "GoToLevelSettings"(w486) -> ()
      }
      frame "CetoniConfigure" {
        n175 = call-dynamic "GetCetoniPump.vi"("object in"=w512, "error in (no error)"=w509) -> ("object out"=w513:refnum<class "Application.lvclass">, "CetoniPump"=w508:refnum<class "CetoniPump.lvclass">, "error out"=w506:errorcluster)  [unwired: 15 in]
        n176 = local read "index"() -> (w504:i32)
        n177 = call-dynamic "ConfigureSyringe.vi"("object in"=w508, "index"=w504, "SyringeSettings"="SyringeSettings", "error in (no error)"=w506) -> ("object out"=w507:refnum<class "CetoniPump.lvclass">, "error out"=w505:errorcluster)  [unwired: 14 in]
        n178 = call-dynamic "SetCetoniPump.vi"("object in"=w513, "CetoniPump"=w507, "error in (no error)"=w505) -> ("object out"=w511:refnum<class "Application.lvclass">, "error out"=w510:errorcluster)  [unwired: 15 in]
      }
      frame "CetoniRefMove" {
        n179 = call-dynamic "GetCetoniPump.vi"("object in"=w525, "error in (no error)"=w522) -> ("object out"=w516:refnum<class "Application.lvclass">, "CetoniPump"=w521:refnum<class "CetoniPump.lvclass">, "error out"=w519:errorcluster)  [unwired: 15 in]
        n180 = call-dynamic "ReferenceMove.vi"("object in"=w521, "index"=0, "error in (no error)"=w519) -> ("object out"=w520:refnum<class "CetoniPump.lvclass">, "error out"=w518:errorcluster)  [unwired: 15 in]
        n181 = call-dynamic "SetCetoniPump.vi"("object in"=w516, "CetoniPump"=w520, "error in (no error)"=w518) -> ("object out"=w524:refnum<class "Application.lvclass">, "error out"=w523:errorcluster)  [unwired: 15 in]
        n182 = call-dynamic "FireStatusEvent.vi"("object in"=w524, "Status"="Reference Move") -> ("object out"=w515:refnum<class "Application.lvclass">)  [unwired: 16 in, 1 out]
      }
      frame "CetoniEmpty" {
        n183 = call-dynamic "GetCetoniPump.vi"("object in"=w534, "error in (no error)"=w531) -> ("object out"=w535:refnum<class "Application.lvclass">, "CetoniPump"=w530:refnum<class "CetoniPump.lvclass">, "error out"=w528:errorcluster)  [unwired: 15 in]
        n184 = local read "index"() -> (w526:i32)
        n185 = call-dynamic "Empty.vi"("object in"=w530, "index"=w526, "error in (no error)"=w528) -> ("object out"=w529:refnum<class "CetoniPump.lvclass">, "error out"=w527:errorcluster)  [unwired: 15 in]
        n186 = call-dynamic "SetCetoniPump.vi"("object in"=w535, "CetoniPump"=w529, "error in (no error)"=w527) -> ("object out"=w533:refnum<class "Application.lvclass">, "error out"=w532:errorcluster)  [unwired: 15 in]
      }
      frame "CetoniMonitor" {
        n187 = call-dynamic "GetCetoniPump.vi"("object in"=w546, "error in (no error)"=w543) -> ("object out"=w547:refnum<class "Application.lvclass">, "CetoniPump"=w542:refnum<class "CetoniPump.lvclass">, "error out"=w540:errorcluster)  [unwired: 15 in]
        n188 = call-dynamic "ReadStatusAllPumps.vi"("object in"=w542, "error in (no error)"=w540) -> ("object out"=w541:refnum<class "CetoniPump.lvclass">, "Array"=→"Array":T5, "error out"=w539:errorcluster)  [unwired: 15 in]
        n189 = local read "Monitor Pump"() -> (w537:bool)
        n190 = call-dynamic "SetCetoniPump.vi"("object in"=w547, "CetoniPump"=w541, "error in (no error)"=w539) -> ("object out"=w545:refnum<class "Application.lvclass">, "error out"=w544:errorcluster)  [unwired: 15 in]
        n191 = case shown="False" w537 {
          tunnel: w545 -> [w548 w551]
          tunnel: [w548 w550] -> w538
          frame False {
          }
          frame True {
            n192 = call-dynamic "EnqueueMain.vi"("object in"=w551, "Message"="CetoniMonitor") -> ("object out"=w550:refnum<class "Application.lvclass">)  [unwired: 16 in, 1 out]
          }
        }
      }
      frame "CetoniStop" {
        n193 = call-dynamic "GetCetoniPump.vi"("object in"=w559, "error in (no error)"=w556) -> ("object out"=w560:refnum<class "Application.lvclass">, "CetoniPump"=w555:refnum<class "CetoniPump.lvclass">, "error out"=w553:errorcluster)  [unwired: 15 in]
        n194 = call-dynamic "StopAllPumps.vi"("object in"=w555, "error in (no error)"=w553) -> ("object out"=w554:refnum<class "CetoniPump.lvclass">, "error out"=w552:errorcluster)  [unwired: 16 in]
        n195 = call-dynamic "SetCetoniPump.vi"("object in"=w560, "CetoniPump"=w554, "error in (no error)"=w552) -> ("object out"=w558:refnum<class "Application.lvclass">, "error out"=w557:errorcluster)  [unwired: 15 in]
      }
      frame "CetoniInit" {
        n196 = case shown="True" "Use Cetoni?" {
          tunnel: w565 -> [w567 w578]
          tunnel: [w567 w569] -> w564
          tunnel: [w566 w576] -> w563
          tunnel: w562 -> [w566 w575]
          frame False {
          }
          frame True {
            n197 = call-dynamic "GetCetoniPump.vi"("object in"=w578, "error in (no error)"=w575) -> ("object out"=w579:refnum<class "Application.lvclass">, "CetoniPump"=w574:refnum<class "CetoniPump.lvclass">, "error out"=w572:errorcluster)  [unwired: 15 in]
            n198 = call "CetoniPump_Init.vi"("object in"=w574, "Device Configuration Path"="Device Configuration Path", "error in (no error)"=w572) -> ("object out"=w573:refnum<class "CetoniPump.lvclass">, "error out"=w571:errorcluster)  [unwired: 15 in]
            n199 = call-dynamic "SetCetoniPump.vi"("object in"=w579, "CetoniPump"=w573, "error in (no error)"=w571) -> ("object out"=w577:refnum<class "Application.lvclass">, "error out"=w576:errorcluster)  [unwired: 15 in]
            n200 = call-dynamic "FireStatusEvent.vi"("object in"=w577, "Status"="Cetoni Initialized") -> ("object out"=w569:refnum<class "Application.lvclass">)  [unwired: 16 in, 1 out]
          }
        }
      }
      frame "AdjustPower" {
        # "Do not adjust if wfg is not enabled, only set it for logging purpose"
        n201 = Variant To Data(type=0.0 ("Desired Power"), Variant=w592) -> (data=w590:dbl)  [unwired: 1 in, 1 out]
        n202 = call-dynamic "FireStatusEvent.vi"("object in"=w600, "Status"="Adjusting Power") -> ("object out"=w594:refnum<class "Application.lvclass">)  [unwired: 16 in, 1 out]
        n203 = call-dynamic "GetInstrumentBase.vi"("object in"=w594, "error in (no error)"=w597) -> ("object out"=w589:refnum<class "Application.lvclass">, "InstrumentBase"=w583:refnum<class "InstrumentBase.lvclass">, "error out"=w588:errorcluster)  [unwired: 15 in]
        n204 = call-dynamic "GetWfgEnabled.vi"("object in"=w583) -> ("object out"=w582:refnum<class "InstrumentBase.lvclass">, "WfgEnabled"=w581:cluster{"Ch1":bool, "Ch2":bool})  [unwired: 16 in, 1 out]
        n205 = Unbundle By Name(w581) -> ("Ch1"=w580:bool)
        n206 = case shown="True" w580 {
          tunnel: w590 -> [w601 w613]
          tunnel: w588 -> [w602 w611]
          tunnel: [w605 w610] -> w586
          tunnel: [_ w609] -> w585
          tunnel: [w603 w607] -> w584
          tunnel: w582 -> [w604 w606]
          frame False {
            n207 = call-dynamic "SetDesiredPower(W).vi"("object in"=w604, "DesiredPower(W)"=w601, "error in (no error)"=w602) -> ("object out"=w605:refnum<class "InstrumentBase.lvclass">, "error out"=w603:errorcluster)  [unwired: 15 in]
          }
          frame True {
            n208 = call-dynamic "AdjustPower.vi"("object in"=w606, "DesiredPower(W)"=w613, "error in (no error)"=w611) -> ("object out"=w612:refnum<class "InstrumentBase.lvclass">, "error out"=w608:errorcluster)  [unwired: 15 in]
            n209 = call-dynamic "GetAmplitudeOk.vi"("object in"=w612, "error in (no error)"=w608) -> ("object out"=w610:refnum<class "InstrumentBase.lvclass">, "AmplitudeOk"=w609:bool, "error out"=w607:errorcluster)  [unwired: 15 in]
          }
        }
        "AmplitudeOk" <- w585
        n210 = call-dynamic "SetInstrumentBase.vi"("object in"=w589, "InstrumentBase"=w586, "error in (no error)"=w584) -> ("object out"=w599:refnum<class "Application.lvclass">, "error out"=w598:errorcluster)  [unwired: 15 in]
        n211 = Wait (ms)(milliseconds to wait=u32 200) -> ()  [unwired: 1 out]
        n212 = call-dynamic "FireStatusEvent.vi"("object in"=w599, "Status"="Power Adjusted") -> ("object out"=w596:refnum<class "Application.lvclass">)  [unwired: 16 in, 1 out]
      }
      frame "Wait" {
        n213 = Variant To Data(Variant=w615) -> (data=w614:dbl)  [unwired: 2 in, 1 out]
        n214 = call-dynamic "Wait.vi"("object in"=w619, "Time Target (s)"=w614, "error in (no error)"=w616) -> ("object out"=w618:refnum<class "Application.lvclass">, "error out"=w617:errorcluster)  [unwired: 15 in]
      }
      frame "WfgConfig" {
        n215 = call-dynamic "GetInstrumentBase.vi"("object in"=w631, "error in (no error)"=w622) -> ("object out"=w630:refnum<class "Application.lvclass">, "InstrumentBase"=w627:refnum<class "InstrumentBase.lvclass">, "error out"=w623:errorcluster)  [unwired: 15 in]
        n216 = call-dynamic "ConfigWFG.vi"("object in"=w627, "Config(var)"=w624, "error in (no error)"=w623) -> ("object out"=w626:refnum<class "InstrumentBase.lvclass">, "error out"=w625:errorcluster)  [unwired: 15 in]
        n217 = call-dynamic "SetInstrumentBase.vi"("object in"=w630, "InstrumentBase"=w626, "error in (no error)"=w625) -> ("object out"=w629:refnum<class "Application.lvclass">, "error out"=w628:errorcluster)  [unwired: 15 in]
        n218 = call-dynamic "FireStatusEvent.vi"("object in"=w629, "Status"="WFG Configured") -> ("object out"=w621:refnum<class "Application.lvclass">)  [unwired: 16 in, 1 out]
      }
      frame "WfgChangeFreq" {
        n219 = Variant To Data(error in=w633, type=T14 {"Ch1.Carrier.Frequency (Hz)"=0.0, "Ch2.Carrier.Frequency (Hz)"=0.0} ("Freq Ch1&2"), Variant=w635) -> (data=w632:T14, error out=w634:errorcluster)
        n220 = call-dynamic "GetInstrumentBase.vi"("object in"=w644, "error in (no error)"=w634) -> ("object out"=w643:refnum<class "Application.lvclass">, "InstrumentBase"=w638:refnum<class "InstrumentBase.lvclass">, "error out"=w640:errorcluster)  [unwired: 15 in]
        n221 = call-dynamic "ChangeFreqWFG.vi"("object in"=w638, "Freq Ch1&2"=w632, "error in (no error)"=w640) -> ("object out"=w637:refnum<class "InstrumentBase.lvclass">, "error out"=w639:errorcluster)  [unwired: 15 in]
        n222 = call-dynamic "SetInstrumentBase.vi"("object in"=w643, "InstrumentBase"=w637, "error in (no error)"=w639) -> ("object out"=w642:refnum<class "Application.lvclass">, "error out"=w641:errorcluster)  [unwired: 15 in]
      }
      frame "WfgEnable" {
        n223 = Variant To Data(error in=w647, type=T13 {"Enable Output WFG Ch1"=TRUE, "Enable Output WFG Ch 2"=TRUE} ("OutputEnable 2"), Variant=w649) -> (data=w646:T13, error out=w648:errorcluster)
        n224 = call-dynamic "GetInstrumentBase.vi"("object in"=w657, "error in (no error)"=w648) -> ("object out"=w656:refnum<class "Application.lvclass">, "InstrumentBase"=w653:refnum<class "InstrumentBase.lvclass">, "error out"=w650:errorcluster)  [unwired: 15 in]
        n225 = call-dynamic "EnableWFGOutput.vi"("object in"=w653, "OutputEnable 2"=w646, "error in (no error)"=w650) -> ("object out"=w652:refnum<class "InstrumentBase.lvclass">, "error out"=w651:errorcluster)  [unwired: 15 in]
        n226 = call-dynamic "SetInstrumentBase.vi"("object in"=w656, "InstrumentBase"=w652, "error in (no error)"=w651) -> ("object out"=w655:refnum<class "Application.lvclass">, "error out"=w654:errorcluster)  [unwired: 15 in]
      }
      frame "MSOConfigure" {
        n227 = call-dynamic "GetInstrumentBase.vi"("object in"=w669, "error in (no error)"=w661) -> ("object out"=w668:refnum<class "Application.lvclass">, "InstrumentBase"=w663:refnum<class "InstrumentBase.lvclass">, "error out"=w665:errorcluster)  [unwired: 15 in]
        n228 = call-dynamic "ConfigMSO.vi"("object in"=w663, "variant"=w660, "error in (no error)"=w665) -> ("object out"=w662:refnum<class "InstrumentBase.lvclass">, "error out"=w664:errorcluster)  [unwired: 15 in]
        n229 = call-dynamic "SetInstrumentBase.vi"("object in"=w668, "InstrumentBase"=w662, "error in (no error)"=w664) -> ("object out"=w667:refnum<class "Application.lvclass">, "error out"=w666:errorcluster)  [unwired: 15 in]
        n230 = call-dynamic "FireStatusEvent.vi"("object in"=w667, "Status"="Configuring MSO") -> ("object out"=w659:refnum<class "Application.lvclass">)  [unwired: 16 in, 1 out]
      }
      frame "MSORead" {
        n231 = call-dynamic "GetInstrumentBase.vi"("object in"=w682, "error in (no error)"=w675) -> ("object out"=w681:refnum<class "Application.lvclass">, "InstrumentBase"=w677:refnum<class "InstrumentBase.lvclass">, "error out"=w679:errorcluster)  [unwired: 15 in]
        n232 = call-dynamic "ReadMSO.vi"("object in"=w677, "error in (no error)"=w679) -> ("object out"=w676:refnum<class "InstrumentBase.lvclass">, "Channels array"=w673:waveform(dbl)[], "error out"=w678:errorcluster)  [unwired: 15 in]
        n233 = call-dynamic "SetInstrumentBase.vi"("object in"=w681, "InstrumentBase"=w676, "error in (no error)"=w678) -> ("object out"=w680:refnum<class "Application.lvclass">, "error out"=w671:errorcluster)  [unwired: 15 in]
        n234 = call-dynamic "FireUIEvent.vi"("object in"=w680, "Message"="UpdateMsoData", "Message Data"=w673, "error in (no error)"=w671) -> ("object out"=w674:refnum<class "Application.lvclass">, "error out"=w670:errorcluster)  [unwired: 14 in]
      }
      frame "MSOAutoRange" {
        n235 = call-dynamic "GetInstrumentBase.vi"("object in"=w700, "error in (no error)"=w695) -> ("object out"=w699:refnum<class "Application.lvclass">, "InstrumentBase"=w690:refnum<class "InstrumentBase.lvclass">, "error out"=w689:errorcluster)  [unwired: 15 in]
        n236 = call-dynamic "AutoRangeMSO.vi"("object in"=w690, "error in (no error)"=w689) -> ("object out"=w688:refnum<class "InstrumentBase.lvclass">, "error out"=w686:errorcluster)  [unwired: 16 in]
        n237 = call-dynamic "ReadMSOConfig.vi"("object in"=w688, "error in (no error)"=w686) -> ("object out"=w687:refnum<class "InstrumentBase.lvclass">, "Config"=w684:T18, "error out"=w685:errorcluster)  [unwired: 15 in]
        n238 = call-dynamic "ReadMSO.vi"("object in"=w687, "error in (no error)"=w685) -> ("object out"=w696:refnum<class "InstrumentBase.lvclass">, "Channels array"=w693:waveform(dbl)[], "error out"=w697:errorcluster)  [unwired: 15 in]
        n239 = call-dynamic "SetInstrumentBase.vi"("object in"=w699, "InstrumentBase"=w696, "error in (no error)"=w697) -> ("object out"=w698:refnum<class "Application.lvclass">, "error out"=w691:errorcluster)  [unwired: 15 in]
        n240 = call-dynamic "FireUIEvent.vi"("object in"=w698, "Message"="UpdateMsoData", "Message Data"=w693, "error in (no error)"=w691) -> ("object out"=w694:refnum<class "Application.lvclass">, "error out"=w683:errorcluster)  [unwired: 14 in]
        n241 = local write "Config"(w684) -> ()
      }
      frame "ScanSaveData" {
        n242 = call-dynamic "SaveData.vi"("object in"=w704, "error in (no error)"=w702) -> ("object out"=w703:refnum<class "Application.lvclass">, "error out"=w701:errorcluster)  [unwired: 16 in]
      }
      frame Default {
        # "'Default' case only runs if there is a message that isn't defined in any of the other cases.  Output a programming error."
        n243 = xnode "Error Ring"("parameter 0"=w706) -> ("error out"=w707:errorcluster)
      }
    }
    n244 = call-dynamic "ErrorHandlerMainLoop.vi"("object in"=w18, "error in (no error)"=w21) -> ("object out"=w19:refnum<class "Application.lvclass">, "error out"=w20:errorcluster)  [unwired: 16 in]
  }
  n245 = while {
    tunnel: [w717] -> w9
    shift-right: [w715] -> _
    shift-left: w4 -> [w720]
    tunnel: w13 -> [w719]
    tunnel: w14 -> [w722]
    stop <- w721 stop-if-true
    # "Event Handling Loop"
    n246 = event shown="[6] <UI Event>: User Event" {
      selector: w722 -> [_ _ _ _ _ _ _ _ _ _ _ _ _ _ _ _ _ _ _ _ _ _ _ _ _ _ _ _ _ _ _ _ _ _ _]
      dyn-events: _ -> [_ _ _ _ _ _ _ _ _ _ _ _ _ _ _ _ _ _ _ _ _ _ _ _ _ _ _ _ _ _ _ _ _ _ _]
      timeout: _ -> [_ _ _ _ _ _ _ _ _ _ _ _ _ _ _ _ _ _ _ _ _ _ _ _ _ _ _ _ _ _ _ _ _ _ _]
      tunnel: [_ _ _ _ _ _ _ _ _ _ _ _ _ _ _ _ _ _ _ _ _ _ _ _ _ _ _ _ _ _ _ _ _ _ TRUE ("Discard?")] -> w721
      tunnel: [w725 w734 w735 w737 w744 w749 w756 w854 w862 w870 w883 w888 w894 w899 w904 w909 w914 w919 w924 w930 w935 w940 w946 w951 w959 w963 w967 w971 w975 w979 w984 w989 w994 w996 w1001] -> w718
      tunnel: w720 -> [w724 w733 w736 w741 w747 w752 w758 w856 w861 w869 w887 w892 w898 w903 w908 w913 w918 w923 w928 w934 w939 w944 w950 w955 w958 w962 w966 w970 w974 w978 w983 w988 w993 w1000 w1002]
      tunnel: [w723 w732 w736 w740 w746 w751 w757 w855 w861 w869 w886 w891 w897 w902 w907 w912 w917 w922 w927 w933 w938 w943 w949 w954 w957 w961 w965 w969 w973 w977 w982 w987 w992 w999 w1002] -> w716
      tunnel: w719 -> [w726 w734 w735 w738 w745 w750 w755 w853 w862 w870 w884 w889 w895 w900 w905 w910 w915 w920 w925 w931 w936 w941 w947 w952 w959 w963 w967 w971 w975 w979 w984 w989 w994 w995 w1001]
      event Panel Close? {
        # "Send the 'Confirm Quit' message if the user closes the panel of the VI. Discard the event so the 'Confirm Quit' message has a chance to run."
        n247 = event-data() -> ()  [unwired: 1 in, 1 out]
        n248 = call-dynamic "EnqueueMain.vi"("object in"=w724, "Message"="Confirm Quit", "error in (no error)"=w726, "Priority Message? (F)"=TRUE) -> ("object out"=w723:refnum<class "Application.lvclass">, "error out"=w725:errorcluster)  [unwired: 14 in]
        n249 = event-data("Discard?"=TRUE) -> ()  [unwired: 1 in, 1 out]
      }
      event "Freq Ch1&2": Value Change {
        n250 = event-data() -> ()  [unwired: 1 in, 2 out]
        n251 = call-dynamic "EnqueueMain.vi"("object in"=w733, "Message"="WfgChangeFreq", "Message Data"="Freq Ch1&2") -> ("object out"=w732:refnum<class "Application.lvclass">)  [unwired: 15 in, 1 out]
      }
      event Application Instance Close {
        # "#CodeRecommended - When a project closes, all VIs within that project are aborted and leave memory. However, any code placed in this event frame is guaranteed to run to completion, so add any cleanup code that absolutely must happen here."
        n252 = event-data() -> ()  [unwired: 1 in, 1 out]
      }
      event "Configure TEC": Value Change {
        n253 = event-data() -> ()  [unwired: 1 in, 2 out]
        n254 = call-dynamic "EnqueueMain.vi"("object in"=w741, "Message"="MeTecConfigure", "error in (no error)"=w738) -> ("object out"=w740:refnum<class "Application.lvclass">, "error out"=w737:errorcluster)  [unwired: 15 in]
      }
      event "Configure MSO": Value Change {
        n255 = event-data() -> ()  [unwired: 1 in, 2 out]
        n256 = call-dynamic "EnqueueMain.vi"("object in"=w747, "Message"="MSOConfigure", "Message Data"="Config", "error in (no error)"=w745) -> ("object out"=w746:refnum<class "Application.lvclass">, "error out"=w744:errorcluster)  [unwired: 14 in]
      }
      event "AutoRange MSO (Volt)": Value Change {
        n257 = event-data() -> ()  [unwired: 1 in, 2 out]
        n258 = call-dynamic "EnqueueMain.vi"("object in"=w752, "Message"="MSOAutoRange", "error in (no error)"=w750) -> ("object out"=w751:refnum<class "Application.lvclass">, "error out"=w749:errorcluster)  [unwired: 15 in]
      }
      event User Event {
        n259 = event-data() -> ("Message"=w754:string, "Message Data"=w753:variant)  [unwired: 1 in]
        n260 = case shown="\"AutoScaleGraph\"" w754 {
          tunnel: w758 -> [w762 w765 w830 w845 w851]
          tunnel: [w762 w763 w830 w845 w851] -> w757
          tunnel: [w761 w764 w828 w834 w849] -> w756
          tunnel: w755 -> [w760 w767 w827 w833 w848]
          tunnel: w753 -> [_ w766 w829 w835 w850]
          frame "False", Default {
            n261 = Merge Errors(errorcluster {"status"=TRUE, "code"=5005, "source"="INvalid String In Message Handling Loop"} ("error in (no error)"), w760) -> (w761:errorcluster)
          }
          frame "UpdateMsoData" {
            n262 = Variant To Data(error in=w767, type=waveform(dbl)[] [{"t0"=timestamp(0 s since 1904-01-01), "dt"=1e-08, "Y"=array[8192 elements]}, {"t0"=timestamp(0 s since 1904-01-01), "dt"=1e-08, "Y"=array[8192 elements]}] ("Waveform Graph"), Variant=w766) -> (data=w775:waveform(dbl)[], error out=w774:errorcluster)
            "MSO Data WaveForms 2" <- w775
            n263 = for {
              tunnel: [w795] -> w773 mode=concatenating
              shift-right: [w790] -> w771
              shift-left: w774 -> [w791]
              tunnel: [w786] -> w772 mode=concatenating
              tunnel: w775 -> [w785] mode=indexing
              i -> [w801]
              n264 = Increment(x=w801) -> (x+1=w796:i32)
              n265 = call-poly <vilib>:"Extract Single Tone Information.vi"("error in (no error)"=w791, "time signal in"=w785) -> ("error out"=w790:errorcluster, "detected phase (deg)"=w787:dbl, "detected amplitude"=w788:dbl, "detected frequency"=w789:dbl)  [unwired: 4 in, 2 out]
              n266 = Number To Decimal String(number=w796) -> (decimal integer string=w802:string)  [unwired: 1 in]
              n267 = Concatenate Strings("Ch" ("string"), w802) -> (w794:string)
              n268 = Concatenate Strings(w794, "Freq") -> (w798:string)
              n269 = Concatenate Strings(w794, "Amp") -> (w797:string)
              n270 = Concatenate Strings(w794, "Phase") -> (w792:string)
              n271 = Build Array(w789, w788, w787) -> (w786:dbl[])
              n272 = Build Array(w798, w797, w792) -> (w795:string[])
            }
            "Data" <- w773
            "V/Hz/Deg" <- w772
            n273 = Index Array(array=w772) -> (element=w768:dbl)  [unwired: 1 in]
            n274 = case shown="True" "AutoScaleCh1" {
              tunnel: w765 -> [w777 w784]
              tunnel: w771 -> [w778 w781]
              tunnel: [w778 w782] -> w764
              tunnel: "AutoScaleGraph" -> [_ w780]
              tunnel: w768 -> [_ w779]
              tunnel: [w777 w783] -> w763
              frame False {
              }
              frame True {
                n275 = call-dynamic "FireUIEvent.vi"("object in"=w784, "Message"=w780, "Message Data"=w779, "error in (no error)"=w781) -> ("object out"=w783:refnum<class "Application.lvclass">, "error out"=w782:errorcluster)  [unwired: 14 in]
              }
            }
          }
          frame "UpdateTempData" {
            # "prevents the waveform chart from loosing history"
            n276 = Variant To Data(error in=w827, type=waveform(dbl)[] [{"t0"=timestamp(0 s since 1904-01-01), "dt"=1.0, "Y"=[]}] ("appended array"), Variant=w829) -> (data=w816:waveform(dbl)[], error out=w828:errorcluster)
            n277 = property on="Waveform Chart" class="WFChart (strict)"() -> ("History Data"=w819:waveform(dbl)[][])  [unwired: 2 in, 2 out]
            n278 = Index Array(array=w816) -> (element #1=w815:waveform(dbl), element #2=w811:waveform(dbl), element #3=w808:waveform(dbl))  [unwired: 3 in]
            n279 = Index Array(array=w816, index=0) -> (element=w818:waveform(dbl))
            n280 = Unbundle By Name(w815) -> ("t0"=w814:timestamp, "Y"=w813:dbl[])
            n281 = Index Array(array=w819, index (col)=0 ("disabled index (col)")) -> (element=w823:waveform(dbl)[])  [unwired: 1 in]
            n282 = Unbundle By Name(w811) -> ("Y"=w810:dbl[])
            n283 = Unbundle By Name(w808) -> ("Y"=w807:dbl[])
            n284 = Index Array(array=w813) -> (element=w812:dbl)  [unwired: 1 in]
            n285 = Index Array(array=w810) -> (element=w809:dbl)  [unwired: 1 in]
            n286 = Unbundle By Name(w818) -> ("t0"=w817:timestamp)
            n287 = Delete From Array(array=w823) -> (deleted portion=w820:waveform(dbl))  [unwired: 2 in, 1 out]
            n288 = Unbundle By Name(w820) -> ("t0"=w822:timestamp)
            n289 = Index Array(array=w807) -> (element=w806:dbl)  [unwired: 1 in]
            n290 = Greater?(x=w817, y=w822) -> (0:w821:bool)
            n291 = case shown="True" w821 {
              tunnel: w816 -> [_ w831]
              frame False {
              }
              frame True {
                "Waveform Chart" <- w831
              }
            }
            n292 = call "rolling buffer.vi"("mem size"="mem size", "Ch2 2"=w806, "Ch2"=w809, "Ch1"=w812, "current time"=w814) -> ("XY Graph"=→"XY Graph":cluster{timestamp[], dbl[]}[])  [unwired: 6 in]
          }
          frame "AutoScaleGraph" {
            n293 = Variant To Data(error in=w833, type=1.0 ("x"), Variant=w835) -> (data=w840:dbl, error out=w834:errorcluster)
            n294 = Divide(x=1.0, y=w840) -> (x/y=w842:dbl)
            n295 = control-ref of="MSO Data WaveForms 2"() -> (w832:refnum<vi>)
            n296 = Multiply(x=5.0, y=w842) -> (x*y=w838:dbl)
            n297 = property on="Property Node" class="WFGraph (strict)"(reference=w832, "XScale.Maximum"=w838) -> ()  [unwired: 1 in, 2 out]
            n298 = property on="Property Node" class="WFGraph (strict)"(reference=w832, "XScale.ScaleFit"=u8 0 ("X Scale.Scale Fit")) -> ()  [unwired: 1 in, 2 out]
            n299 = property on="Property Node" class="WFGraph (strict)"(reference=w832, "XScale.Minimum"=0.0 ("X Scale.Range:Maximum")) -> ()  [unwired: 1 in, 2 out]
            n300 = property on="Property Node" class="WFGraph (strict)"(reference=w832, "YScale.ScaleFit"=u8 1 ("Y Scale.Scale Fit")) -> ()  [unwired: 1 in, 2 out]
          }
          frame "UpdateStatus" {
            n301 = Variant To Data(error in=w848, type="", Variant=w850) -> (data=→"Status":string, error out=w849:errorcluster)
          }
        }
      }
      event "Start Experiment": Value Change {
        n302 = event-data() -> ()  [unwired: 1 in, 6 out]
        n303 = call-dynamic "EnqueueMain.vi"("object in"=w856, "Message"="StartExperiment", "error in (no error)"=w853) -> ("object out"=w855:refnum<class "Application.lvclass">, "error out"=w854:errorcluster)  [unwired: 15 in]
      }
      event "Fill List": Value Change {
        n304 = event-data() -> ()  [unwired: 1 in, 6 out]
        n305 = for {
          N: "Number of Frequencies" -> [_]
          tunnel: "Freq Start" -> [w864]
          tunnel: "Freq Increment" -> [w866]
          tunnel: [w863] -> w857 mode=indexing
          i -> [w867]
          n306 = Multiply(x=w866, y=w867) -> (x*y=w865:dbl)
          n307 = Add(x=w864, y=w865) -> (x+y=w863:dbl)
        }
        n308 = local write "List of Frequencies (Hz)"(w857) -> ()
      }
      event "Chart Length": Value Change {
        n309 = event-data() -> ()  [unwired: 1 in, 6 out]
        n310 = case shown="\"1 h\"" "Chart Length" {
          frame "60 s", Default {
            n311 = Get Date/Time In Seconds() -> (seconds since 1Jan1904=w874:timestamp)
            n312 = Subtract(x=w874, y=60.0) -> (x-y=w873:timestamp)
            n313 = To Double Precision Float(number=w873) -> (double precision float=w872:dbl)
            n314 = property on="Waveform Chart" class="WFChart (strict)"("XScale.Minimum"=w872) -> ()  [unwired: 2 in, 2 out]
          }
          frame "10 minutes" {
            n315 = Get Date/Time In Seconds() -> (seconds since 1Jan1904=w878:timestamp)
            n316 = Subtract(x=w878, y=600.0) -> (x-y=w876:timestamp)
            n317 = To Double Precision Float(number=w876) -> (double precision float=w875:dbl)
            n318 = property on="Waveform Chart" class="WFChart (strict)"("XScale.Minimum"=w875) -> ()  [unwired: 2 in, 2 out]
          }
          frame "1 h" {
            n319 = Get Date/Time In Seconds() -> (seconds since 1Jan1904=w882:timestamp)
            n320 = Subtract(x=w882, y=3600.0) -> (x-y=w880:timestamp)
            n321 = To Double Precision Float(number=w880) -> (double precision float=w879:dbl)
            n322 = property on="Waveform Chart" class="WFChart (strict)"("XScale.Minimum"=w879) -> ()  [unwired: 2 in, 2 out]
          }
        }
      }
      event "Read MSO": Value Change {
        n323 = event-data() -> ()  [unwired: 1 in, 2 out]
        n324 = call-dynamic "EnqueueMain.vi"("object in"=w887, "Message"="MSORead", "error in (no error)"=w884) -> ("object out"=w886:refnum<class "Application.lvclass">, "error out"=w883:errorcluster)  [unwired: 15 in]
      }
      event "ABORT": Value Change {
        n325 = event-data() -> ()  [unwired: 1 in, 2 out]
        n326 = call-dynamic "EnqueueMain.vi"("object in"=w892, "Message"="Abort", "error in (no error)"=w889) -> ("object out"=w891:refnum<class "Application.lvclass">, "error out"=w888:errorcluster)  [unwired: 15 in]
      }
      event "AdjustPower": Value Change {
        n327 = event-data() -> ()  [unwired: 1 in, 2 out]
        n328 = call-dynamic "EnqueueMain.vi"("object in"=w898, "Message"="AdjustPower", "Message Data"="DesiredPower(W)", "error in (no error)"=w895) -> ("object out"=w897:refnum<class "Application.lvclass">, "error out"=w894:errorcluster)  [unwired: 14 in]
      }
      event "MeasurePower": Value Change {
        n329 = event-data() -> ()  [unwired: 1 in, 2 out]
        n330 = call-dynamic "EnqueueMain.vi"("object in"=w903, "Message"="MeasurePwr", "error in (no error)"=w900) -> ("object out"=w902:refnum<class "Application.lvclass">, "error out"=w899:errorcluster)  [unwired: 15 in]
      }
      event "Refill": Value Change {
        n331 = event-data() -> ()  [unwired: 1 in, 2 out]
        n332 = call-dynamic "EnqueueMain.vi"("object in"=w908, "Message"="CetoniRefill", "error in (no error)"=w905) -> ("object out"=w907:refnum<class "Application.lvclass">, "error out"=w904:errorcluster)  [unwired: 15 in]
      }
      event "ReferenceMove": Value Change {
        n333 = event-data() -> ()  [unwired: 1 in, 2 out]
        n334 = call-dynamic "EnqueueMain.vi"("object in"=w913, "Message"="CetoniRefMove", "error in (no error)"=w910) -> ("object out"=w912:refnum<class "Application.lvclass">, "error out"=w909:errorcluster)  [unwired: 15 in]
      }
      event "Conditional Refill": Value Change {
        n335 = event-data() -> ()  [unwired: 1 in, 2 out]
        n336 = call-dynamic "EnqueueMain.vi"("object in"=w918, "Message"="CetoniCondRefill", "error in (no error)"=w915) -> ("object out"=w917:refnum<class "Application.lvclass">, "error out"=w914:errorcluster)  [unwired: 15 in]
      }
      event "Empty": Value Change {
        n337 = event-data() -> ()  [unwired: 1 in, 2 out]
        n338 = call-dynamic "EnqueueMain.vi"("object in"=w923, "Message"="CetoniEmpty", "error in (no error)"=w920) -> ("object out"=w922:refnum<class "Application.lvclass">, "error out"=w919:errorcluster)  [unwired: 15 in]
      }
      event "Configure Syringe": Value Change {
        n339 = event-data() -> ()  [unwired: 1 in, 2 out]
        n340 = call-dynamic "EnqueueMain.vi"("object in"=w928, "Message"="CetoniConfigure", "error in (no error)"=w925) -> ("object out"=w927:refnum<class "Application.lvclass">, "error out"=w924:errorcluster)  [unwired: 15 in]
      }
      event "ValveControl.Valve Position": Value Change {
        n341 = event-data() -> ()  [unwired: 1 in, 2 out]
        n342 = call-dynamic "EnqueueMain.vi"("object in"=w934, "Message"="CetoniToggleValve", "Message Data"="ValveControl", "error in (no error)"=w931) -> ("object out"=w933:refnum<class "Application.lvclass">, "error out"=w930:errorcluster)  [unwired: 14 in]
      }
      event "Stop pumps": Value Change {
        n343 = event-data() -> ()  [unwired: 1 in, 2 out]
        n344 = call-dynamic "EnqueueMain.vi"("object in"=w939, "Message"="CetoniStop", "error in (no error)"=w936) -> ("object out"=w938:refnum<class "Application.lvclass">, "error out"=w935:errorcluster)  [unwired: 15 in]
      }
      event "Monitor Pump": Value Change {
        n345 = event-data() -> ()  [unwired: 1 in, 2 out]
        n346 = call-dynamic "EnqueueMain.vi"("object in"=w944, "Message"="CetoniMonitor", "error in (no error)"=w941) -> ("object out"=w943:refnum<class "Application.lvclass">, "error out"=w940:errorcluster)  [unwired: 15 in]
      }
      event "Go to Level": Value Change {
        n347 = event-data() -> ()  [unwired: 1 in, 2 out]
        n348 = call-dynamic "EnqueueMain.vi"("object in"=w950, "Message"="CetoniGoToLevel", "Message Data"="GoToLevelSettings", "error in (no error)"=w947) -> ("object out"=w949:refnum<class "Application.lvclass">, "error out"=w946:errorcluster)  [unwired: 14 in]
      }
      event "Run Power Scan": Value Change {
        n349 = event-data() -> ()  [unwired: 1 in, 2 out]
        n350 = call-dynamic "EnqueueMain.vi"("object in"=w955, "Message"="StartPwrScan", "error in (no error)"=w952) -> ("object out"=w954:refnum<class "Application.lvclass">, "error out"=w951:errorcluster)  [unwired: 15 in]
      }
      event "Monitor": Value Change {
        n351 = event-data() -> ()  [unwired: 1 in, 2 out]
        n352 = call-dynamic "EnqueueMain.vi"("object in"=w958, "Message"="MeTecMonitor") -> ("object out"=w957:refnum<class "Application.lvclass">)  [unwired: 16 in, 1 out]
      }
      event "Metec Flush Memory": Value Change {
        n353 = event-data() -> ()  [unwired: 1 in, 2 out]
        n354 = call-dynamic "EnqueueMain.vi"("object in"=w962, "Message"="MeTecFlush") -> ("object out"=w961:refnum<class "Application.lvclass">)  [unwired: 16 in, 1 out]
      }
      event "ResetMtec": Value Change {
        n355 = event-data() -> ()  [unwired: 1 in, 2 out]
        n356 = call-dynamic "EnqueueMain.vi"("object in"=w966, "Message"="MeTecReset") -> ("object out"=w965:refnum<class "Application.lvclass">)  [unwired: 16 in, 1 out]
      }
      event "Initialize System": Value Change {
        n357 = event-data() -> ()  [unwired: 1 in, 2 out]
        n358 = call-dynamic "EnqueueMain.vi"("object in"=w970, "Message"="Initialize") -> ("object out"=w969:refnum<class "Application.lvclass">)  [unwired: 16 in, 1 out]
      }
      event "Image": Value Change {
        n359 = event-data() -> ()  [unwired: 1 in, 2 out]
        n360 = call-dynamic "EnqueueMain.vi"("object in"=w974, "Message"="HamamatsuImage") -> ("object out"=w973:refnum<class "Application.lvclass">)  [unwired: 16 in, 1 out]
      }
      event "Configure": Value Change {
        n361 = event-data() -> ()  [unwired: 1 in, 2 out]
        n362 = call-dynamic "EnqueueMain.vi"("object in"=w978, "Message"="HamamatsuConfigure") -> ("object out"=w977:refnum<class "Application.lvclass">)  [unwired: 16 in, 1 out]
      }
      event "Config WFG": Value Change {
        n363 = event-data() -> ()  [unwired: 1 in, 2 out]
        n364 = call-dynamic "EnqueueMain.vi"("object in"=w983, "Message"="WfgConfig", "Message Data"="Configdatastd") -> ("object out"=w982:refnum<class "Application.lvclass">)  [unwired: 15 in, 1 out]
      }
      event "Configdatastd": Value Change {
        n365 = event-data() -> ()  [unwired: 1 in, 2 out]
        n366 = local read "Configdatastd"() -> (w985:T15)
        n367 = call-dynamic "EnqueueMain.vi"("object in"=w988, "Message"="WfgConfig", "Message Data"=w985) -> ("object out"=w987:refnum<class "Application.lvclass">)  [unwired: 15 in, 1 out]
      }
      event "OutputEnable": Value Change {
        n368 = event-data() -> ()  [unwired: 1 in, 2 out]
        n369 = call-dynamic "EnqueueMain.vi"("object in"=w993, "Message"="WfgEnable", "Message Data"="OutputEnable") -> ("object out"=w992:refnum<class "Application.lvclass">)  [unwired: 15 in, 1 out]
      }
      event "Exit": Value Change {
        n370 = event-data() -> ()  [unwired: 1 in, 1 out]
        n371 = call-dynamic "EnqueueMain.vi"("object in"=w1000, "Message"="Exit", "Message Data"=w995, "error in (no error)"=w995, "Priority Message? (F)"=TRUE) -> ("object out"=w999:refnum<class "Application.lvclass">, "error out"=w996:errorcluster)  [unwired: 13 in]
      }
      event User Event {
        (unwired) "\"Exit\" button pressed" ("VI Stopped")
        # "The Message Handling Loop processed an \"Exit\" message, which fired this event to stop the Event Handling Loop."
        n372 = event-data() -> ()  [unwired: 1 in, 1 out]
      }
    }
    n373 = call-dynamic "ErrorHandlerEventLoop.vi"("object in"=w716, "error in (no error)"=w718) -> ("object out"=w715:refnum<class "Application.lvclass">, "error out"=w717:errorcluster)  [unwired: 16 in]
  }
  n374 = Merge Errors(w9, w10) -> (w8:errorcluster)
  n375 = call-dynamic "CleanUp.vi"("object in"=w11, "error in (no error)"=w8) -> ("error out"=→"error out":errorcluster)  [unwired: 16 in, 1 out]
